vi "MegaAwesome_9_12_12a_JW.vi"() -> ()   [LabVIEW 2011]
uses:
  MegaAwesome_States.ctl
  <vilib>/Utility/file.llb/Read From Spreadsheet File (string).vi
  <vilib>/Utility/file.llb/Write To Spreadsheet File (string).vi
panel:
  in  "Slider Min":dbl=5.0
  in  "Slider Max":dbl=5.0
  out "Opj X Axis":string
  out "X Axis Display Type":string
  in  "Index-Sat":dbl=5.0
  in  "Index-Lin":dbl=5.0
  in  "IndexLog-Lin":dbl=5.0
  in  "IndexLog-Sat":dbl=5.0 caption="Num Pts"
  out "Lin Id-Log Used":dbl[](array[numeric])
  out "Lin-Vg Array-Log Used":dbl[](array[numeric])
  out "Total Width":dbl
  in  "New: Comments":string
  out "Save Array":string[][](array[string])
  out "Folder Index":i32 caption="Length"
  out "Sat Id-Used":dbl[](array[numeric])
  out "Sat Vg Array-Used":dbl[](array[numeric])
  out "Vg Array-Log-Used":dbl[](array[numeric])
  out "Sat Id-Log-Used":dbl[](array[numeric])
  out "Lin Id-Used":dbl[](array[numeric])
  out "Lin-Vg Array-Used":dbl[](array[numeric])
  out "Lin Vd":dbl
  out "Recorded Prop":T1
  out "Current State":T2
  in  "Main Tab Control":T3(tab)
  in  "Image Folder":path
  out "Image File":path=path "D:/UserData/Desktop/Jeremy/WFU/Research/Programs/VI mods/Image Not Found.png"
  in  "Transfer File":path
  out "Transfer Folder":path
  out "Fabrication Prop":T4
  in  "Transport ?":bool
  in  "Transfer Plots":T5(tab)=enum."Saturation"
  in  "Lin-Trans Slider":dbl(slide) step=1.0 scale=-40.0..40.0 scale format="%#_1p"
  out "Sqrt-Lin":cluster{dbl[], dbl[]}[](graph)
  in  "Sat-Trans Slider":dbl(slide) step=1.0 scale=-40.0..40.0 scale format="%#_1p"
  out "Sqrt-Sat":cluster{dbl[], dbl[]}[](graph)
  out "Raw- Lin":cluster{dbl[], dbl[]}[](graph)
  out "Raw- Sat":cluster{dbl[], dbl[]}[](graph)
  in  "Log Plots":enum32{"Linear", "Saturation", "Transport"}(tab)=enum."Saturation"
  in  "Lin-Log Slider":dbl(slide) step=1.0 scale=-40.0..40.0 scale format="%#_1p"
  out "Log-Lin":cluster{dbl[], dbl[]}[](graph)
  in  "Sat-Log Slider":dbl(slide) step=1.0 scale=-40.0..40.0 scale format="%#_1p"
  out "Sat-Log":cluster{dbl[], dbl[]}[](graph)
  out "Transport":cluster{dbl[], dbl[]}[](graph)
  in  "Manual Controls":T6
  in  "File Controls":T7
  out "Date Recorded":string="Date Recorded" caption="Measured"
  out "Data Name:":string
  out "Image Name":string
  out "Index":string
  out "Date Created":string caption="Fabricated"
  in  "Comments:":string
  out "Rec: Length":dbl caption="Length" format="%#_3g"
  out "Rec: Width":dbl caption="Width" format="%#_4g"
  out "Rec: Dielectric (d)":dbl caption="Dielectric (d)" format="%#_3g"
  in  "New: Dielectric":dbl
  in  "New: Length":dbl
  in  "New: Width":dbl
  out "Rec: Temp":dbl caption="Sample Temp" format="%.1f"
  in  "New: Temp":dbl format="%.1f"
  out "Image Out":T8(plugin-control)
  in  "Num Pts":dbl=5.0
  in  "Num Pts Log":dbl=5.0 caption="Num Pts"
  out "Recorded Values Cluster":T9
  out "Calculated Values Cluster":T9 caption="Recorded Values Cluster"
  out "Re-Calculated Values Cluster":T9 caption="Recorded Values Cluster"
  in  "Independant Variable:":string(combo)="Length (um):"
  out "Image Preview":T8(plugin-control)
  in  "No Image File":path=path "\\\\acad1\\physics/Jurchescu-group/JW-PD/Mega Awesome/Image Not Found.png"
  in  "Room Temp":dbl=294.0
  in  "Origin Project File":path=path "\\\\acad1\\physics/Jurchescu-group/JW-PD/Group Library/Origin Project Files/DeviceData_8_10_12a_JW.opj"
  in  "Transport Style Controls":T10={"Transport Line Size"=1, "Transport Line Color"=16772608} {"Transport Line Size" items=["Extra Small", "Small", "Medium", "Large", "Extra Large"]}
  # "Image Location"
  # "Recorded"
  # "Calculated"
  # "Re-Calculated"
  # "Manual"
  # "Used points display at y=0\nValues are wrong w/ slider"
  # "Slider\nDoesn't\nWork"
  # "Slider\nDoesn't\nWork"
  # "No new points displayed"
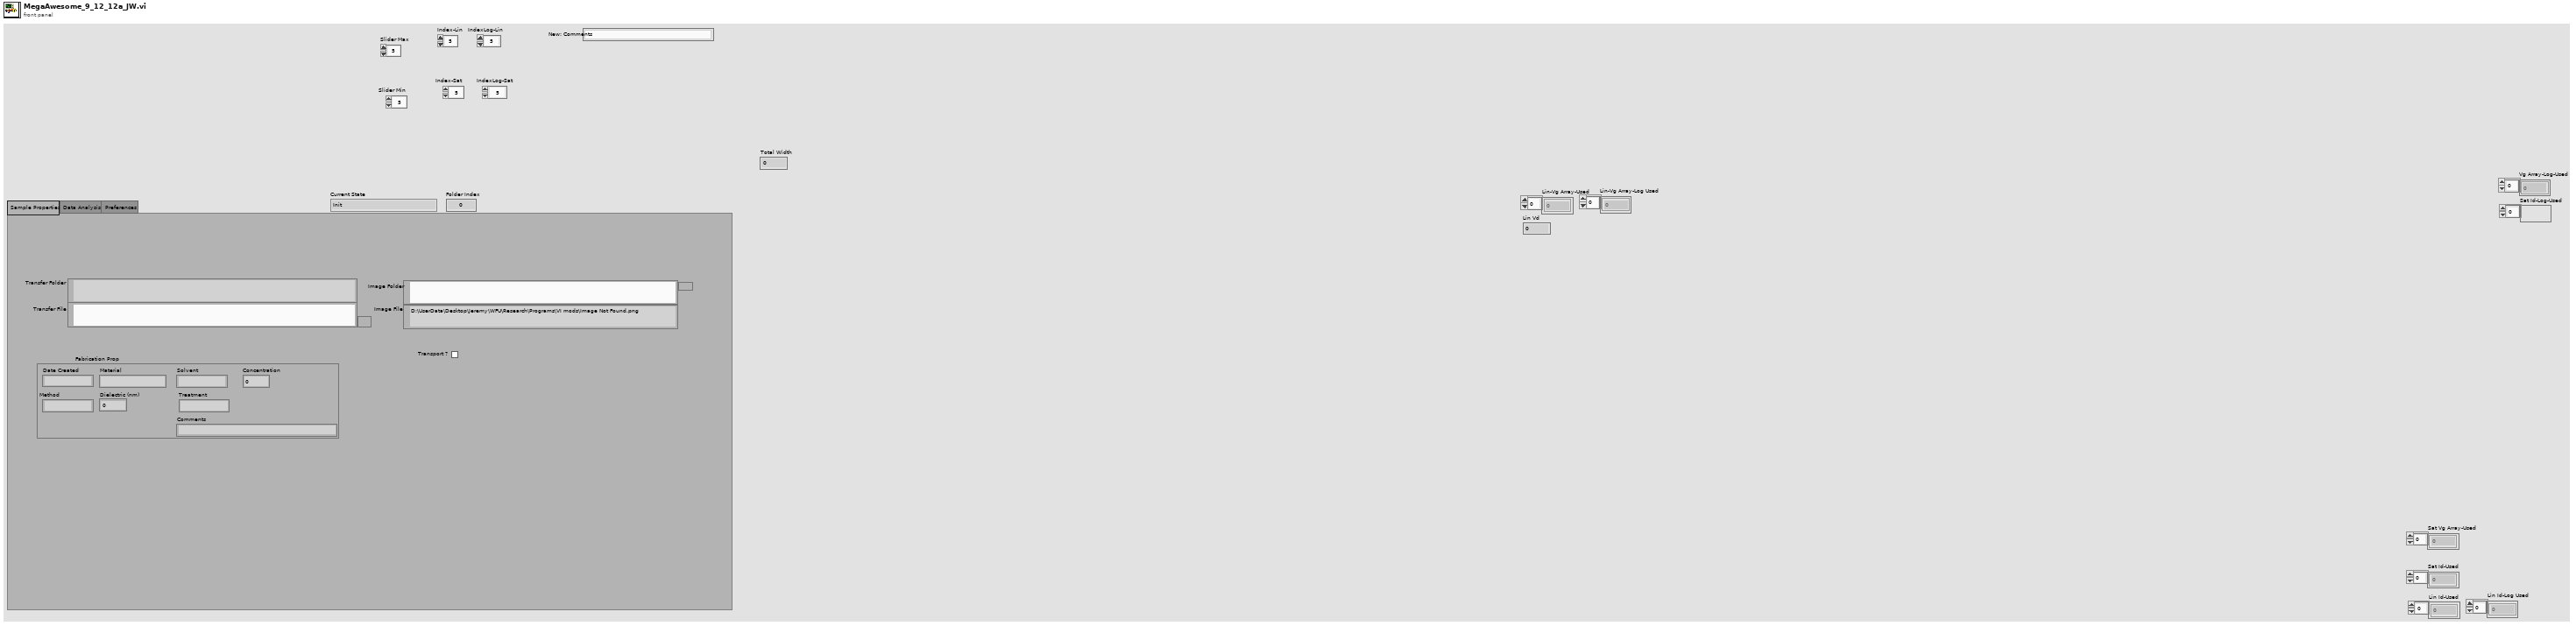
[diagram p1: front panel]
types:
  T1 = cluster{"Date Recorded":string, "Index":string, "Length":dbl, "Width":dbl, "Sample Temp":dbl}
  T2 = typedef "MegaAwesome_States.ctl" = enum16{"Init", "File Missing", "No Event", "Read Data", "Calculated Values", "Re-Calculated Values", "Next File", "Previous File", "Discard File", "Save", "Save Lines", "Export", "Exit"}
  T3 = enum32{"Sample Properties", "Data Analysis", "Preferences"}
  T4 = cluster{"Date Created":string, "Material":string, "Solvent":string, "Concentration":dbl, "Method":string, "Dielectric (nm)":dbl, "Treatment":string, "Comments":string}
  T5 = enum32{"Linear", "Saturation", "Raw-Linear", "Raw-Saturation"}
  T6 = cluster{"Manual-Temp":bool, "Manual-Width":bool, "Manuel-Length":bool, "Manuel-Dielectric":bool, "Manual Comments":bool}
  T7 = cluster{"Previous File":bool, "Discard ":bool, "Save Lines":bool, "Close":bool, "Next File ":bool, "Save":bool, "Save Next":bool, "Export":bool}
  T8 = typedef "IMAQ Image.ctl" = refnum<image>
  T9 = cluster{"Mobility-Sat":dbl, "Moblitity-Lin":dbl, "On/Off":dbl, "Off Current":dbl, "Vt-Sat":dbl, "STS":dbl, "Trap Density-VT":dbl, "Trap Density-STS":dbl}
  T10 = cluster{"Transport Line Size":u16, "Transport Line Color":u32}
  T11 = cluster{"[0]":cluster{dbl[], dbl[]}, "[1]":cluster{dbl[], dbl[]}, "[2]":cluster{dbl[], dbl[]}, "[3]":cluster{dbl[], dbl[]}, "[4]":cluster{dbl[], dbl[]}, "[5]":cluster{dbl[], dbl[]}, "[6]":cluster{dbl[], dbl[]}, "[7]":cluster{dbl[], dbl[]}, "[8]":cluster{dbl[], dbl[]}}
  T12 = cluster{"Sat Vg Used":dbl[], "Sat Sqrt(Id) Used ":dbl[], "Lin Vg Used":dbl[], "Lin Sqrt(Id) Used":dbl[], "Index-Lin":dbl, "Index-Sat":dbl}
  T13 = cluster{"Raw Sat":cluster{dbl[], dbl[]}[], "Sqrt Sat":cluster{dbl[], dbl[]}[], "Log Sat":cluster{dbl[], dbl[]}[], "Raw Lin":cluster{dbl[], dbl[]}[], "Sqrt Lin":cluster{dbl[], dbl[]}[], "Log Lin":cluster{dbl[], dbl[]}[]}
  T14 = cluster{"Mobility-Sat":dbl, "Vt-Sat":dbl, "Mobility-Lin":dbl, "Vt-Lin":dbl, "Off I-Sat":dbl, "On/Off I-Sat":dbl}
  T15 = cluster{"Sat Vg Used":dbl[], "Sat Log(Id) Used":dbl[], "Lin Vg Used":dbl[], "Lin Log(Id) Used":dbl[], "STS Index-Sat":dbl, "STS Index-Lin":dbl}
  T16 = cluster{"Independant  Variable Indicator":string, "Parameter String Indicator":string}
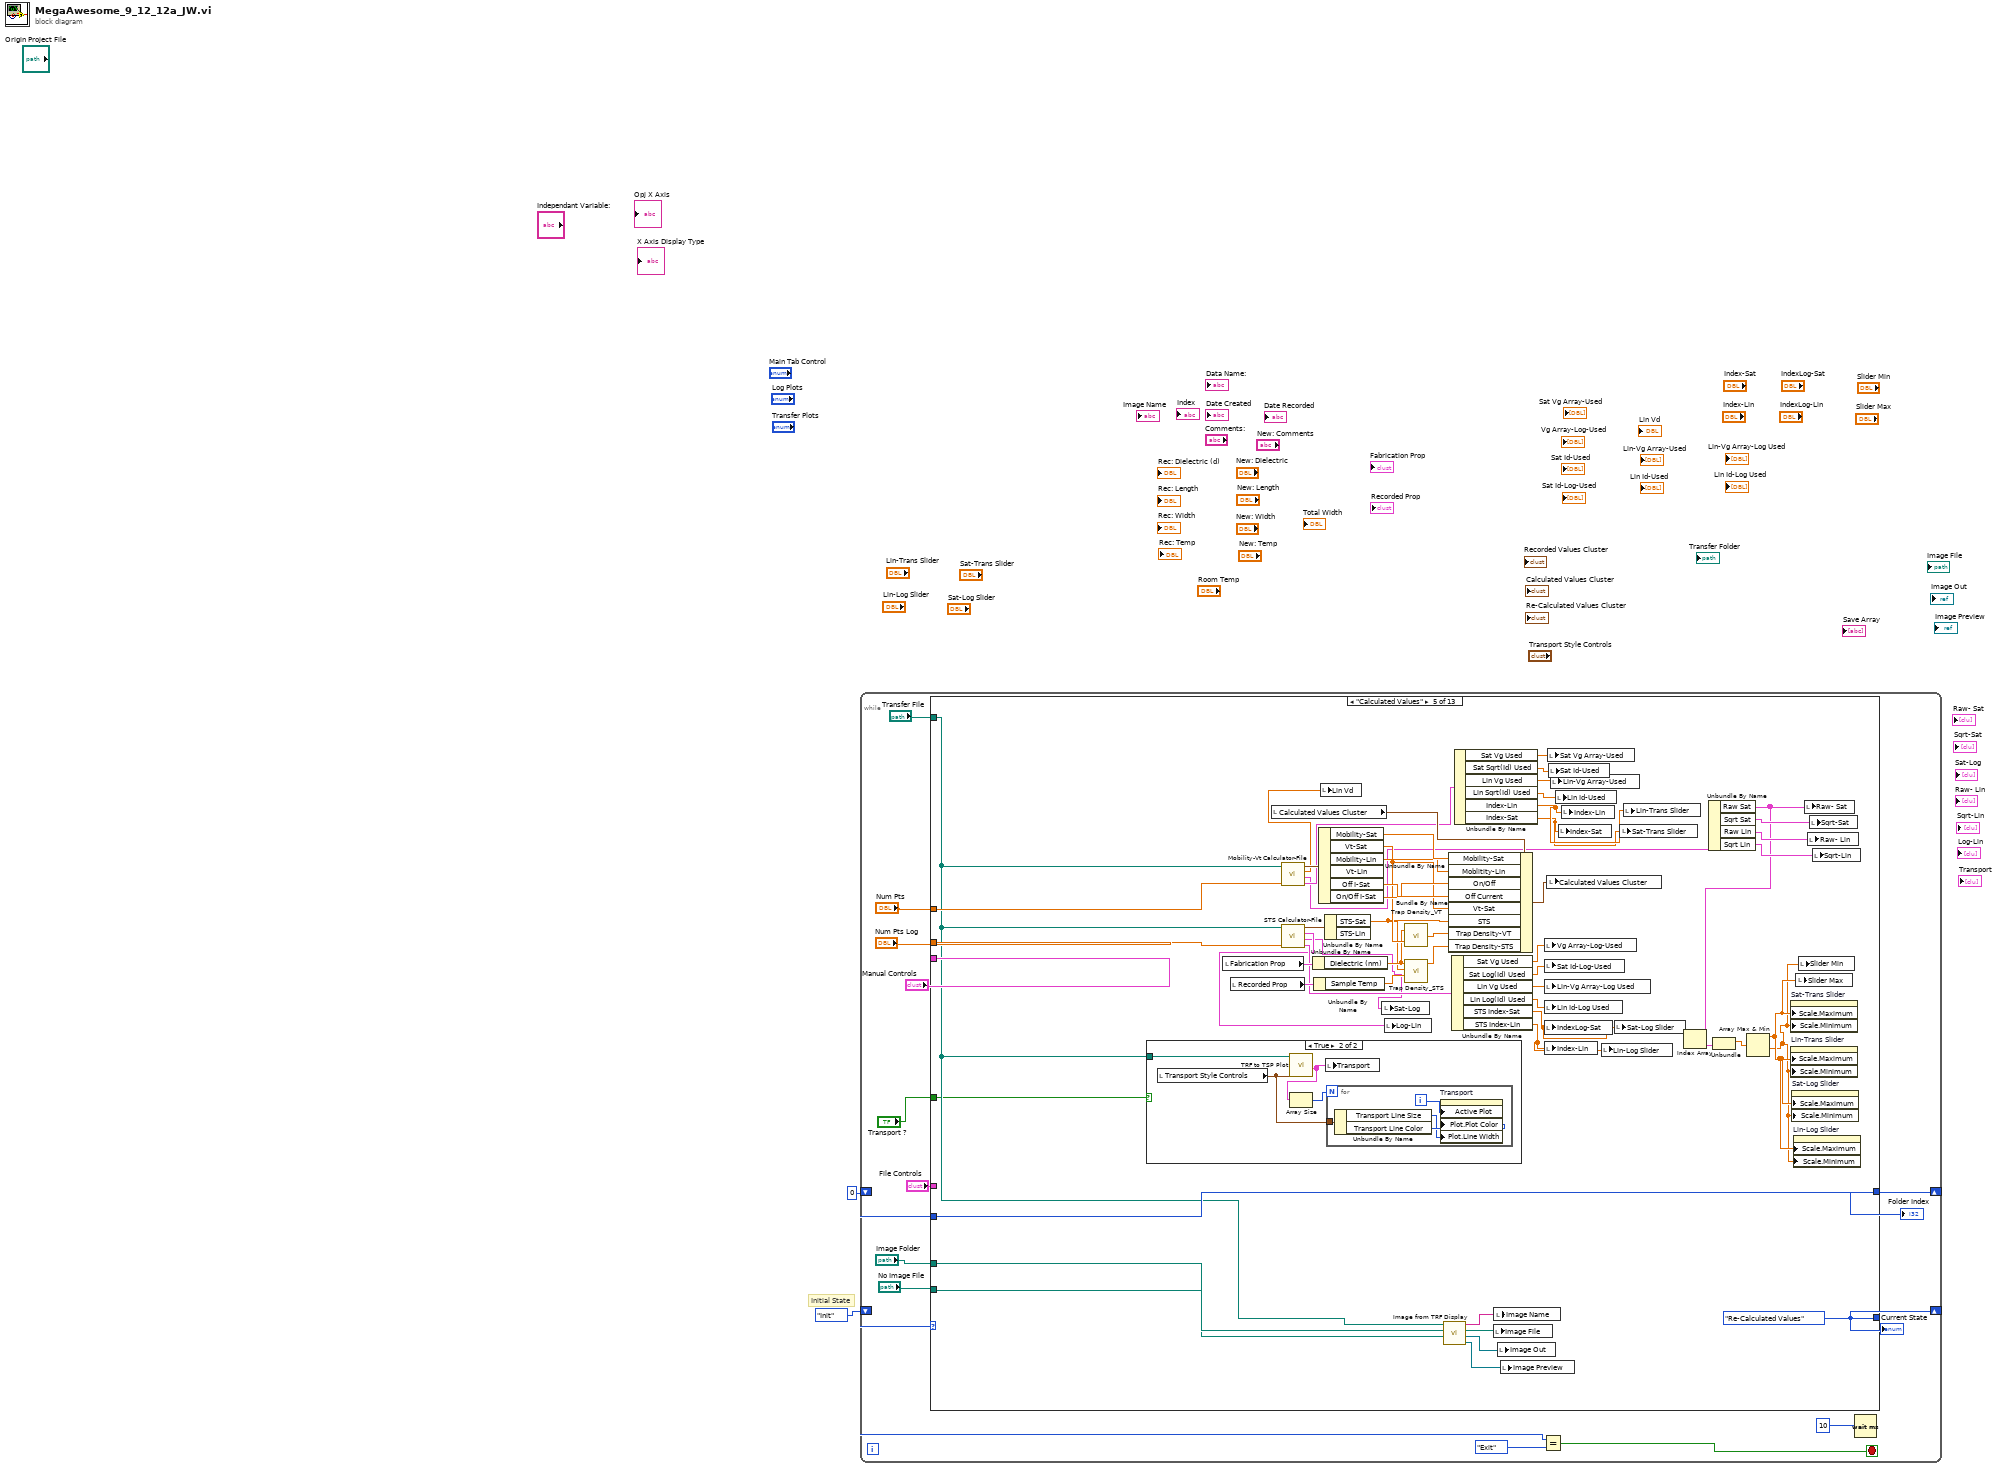
[diagram p0: block diagram]
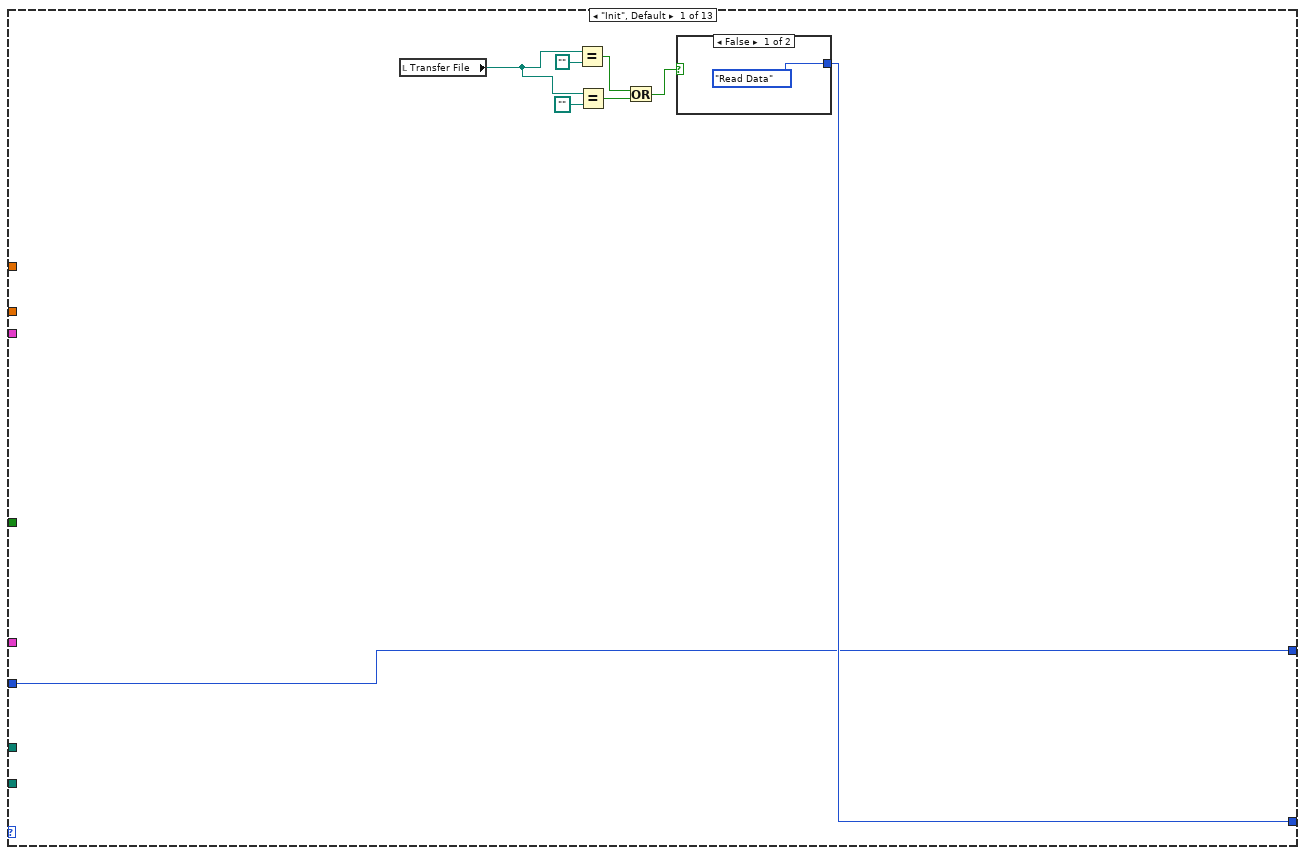
[diagram p2: hidden frame]
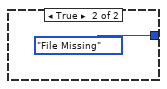
[diagram p3: hidden frame]
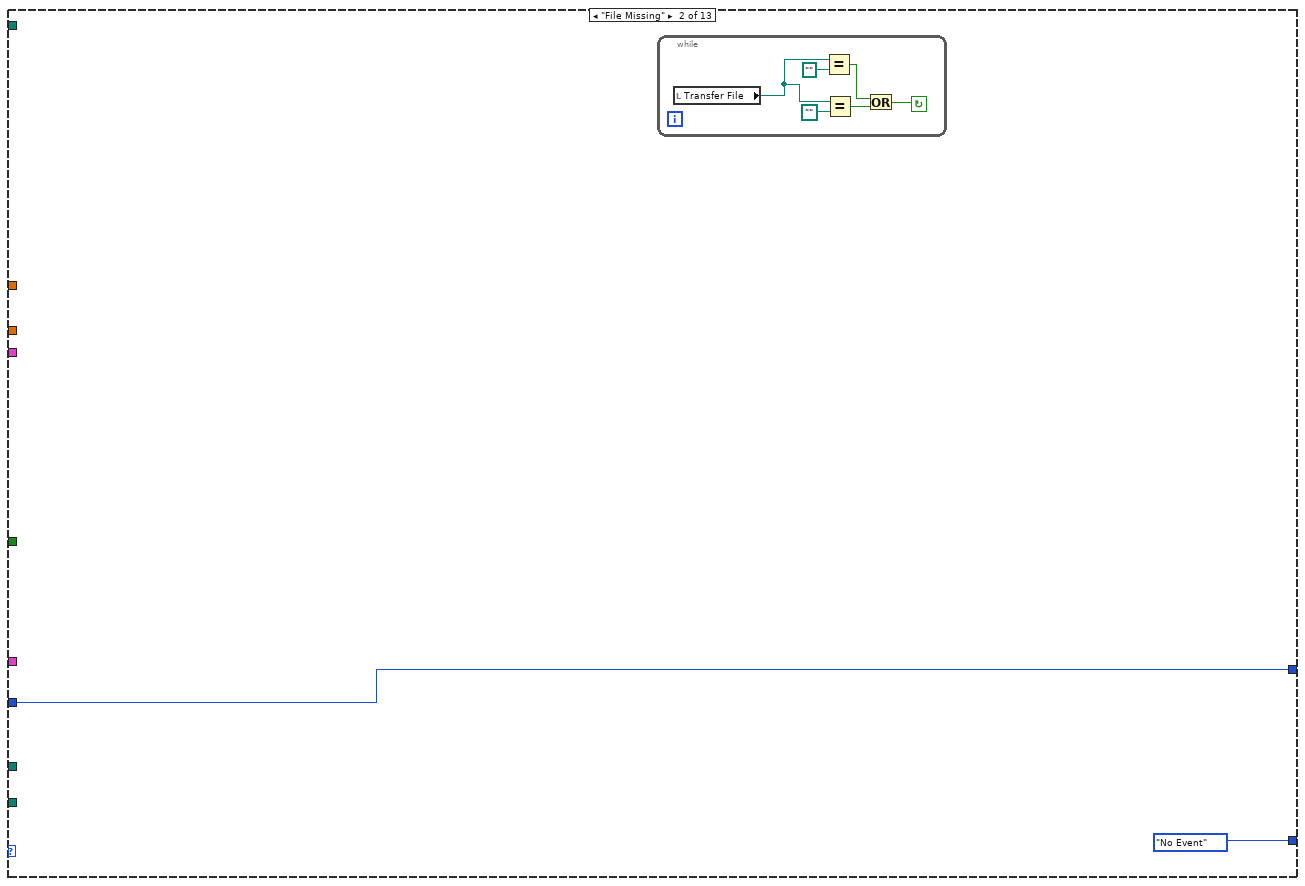
[diagram p4: hidden frame]
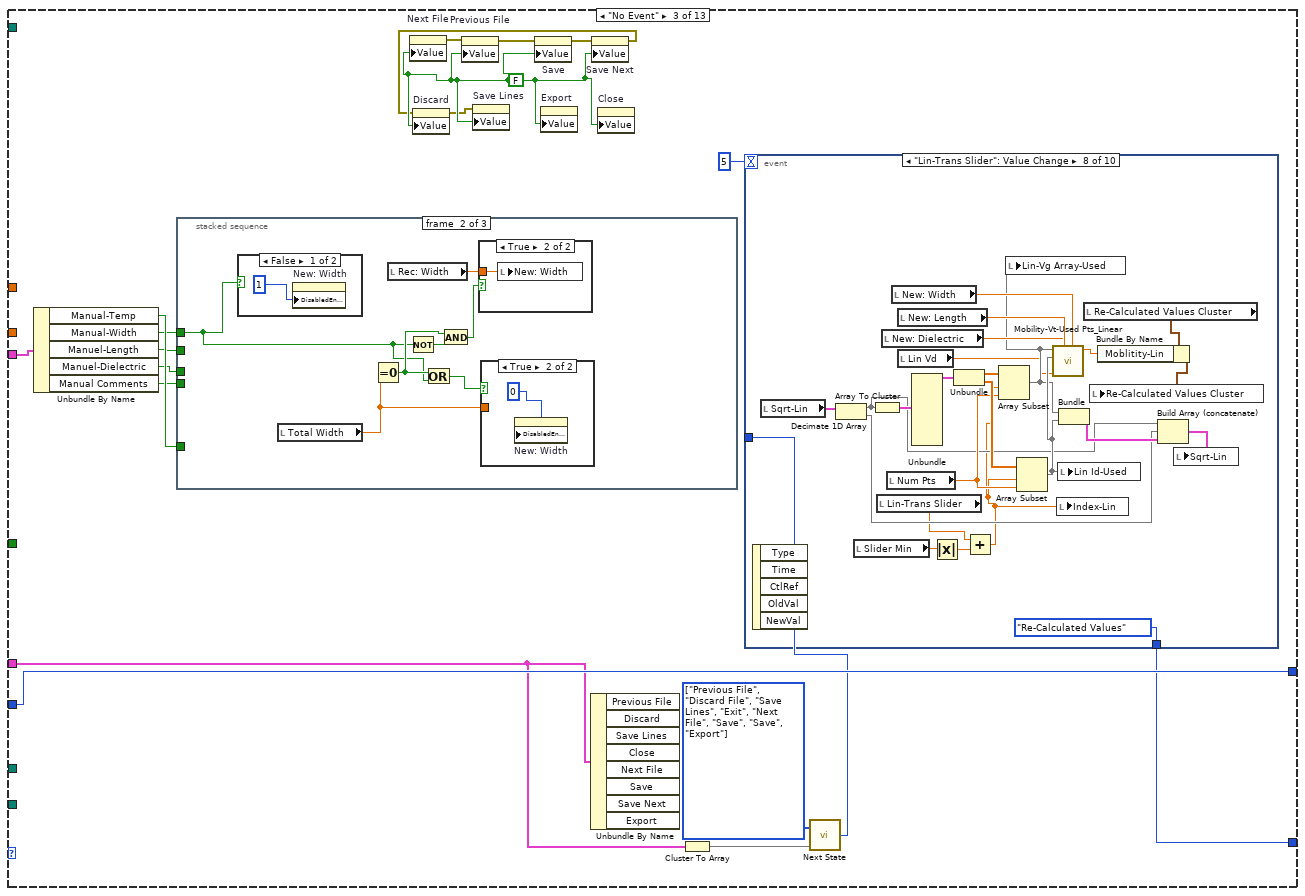
[diagram p5: hidden frame]
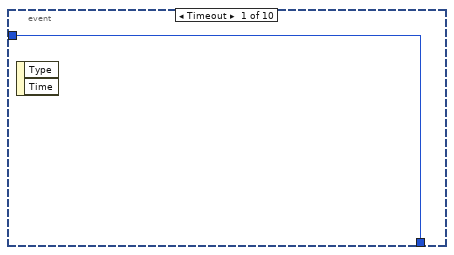
[diagram p6: hidden frame]
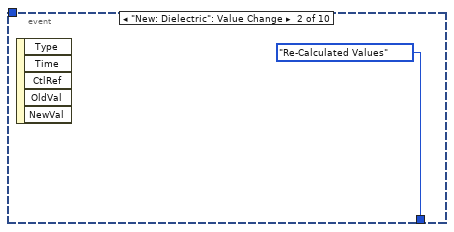
[diagram p7: hidden frame]
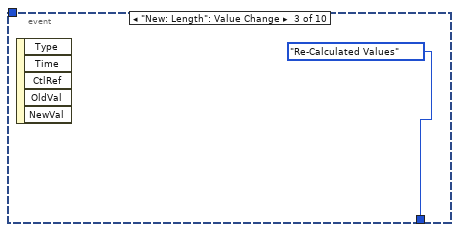
[diagram p8: hidden frame]
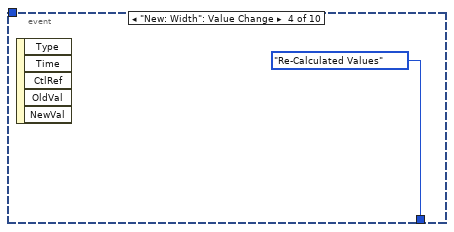
[diagram p9: hidden frame]
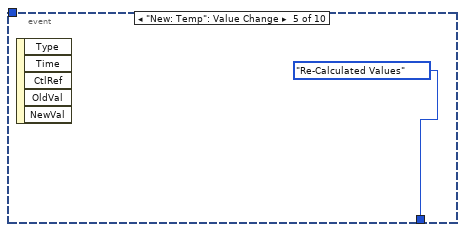
[diagram p10: hidden frame]
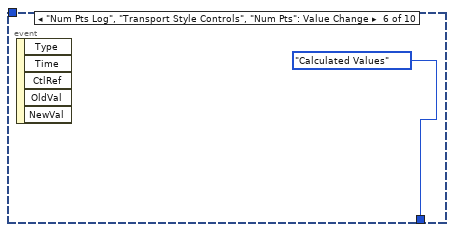
[diagram p11: hidden frame]
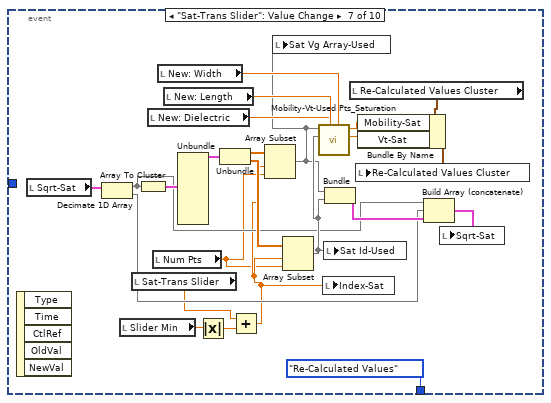
[diagram p12: hidden frame]
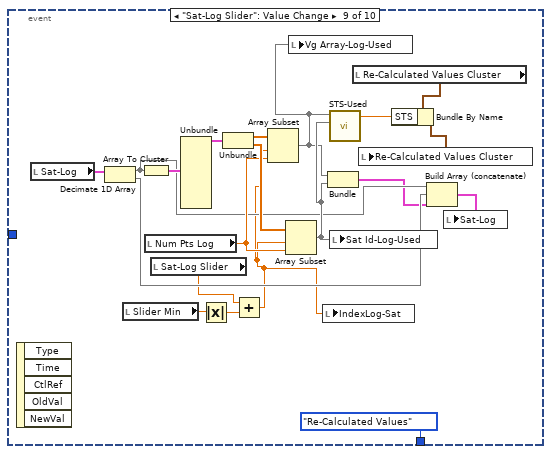
[diagram p13: hidden frame]
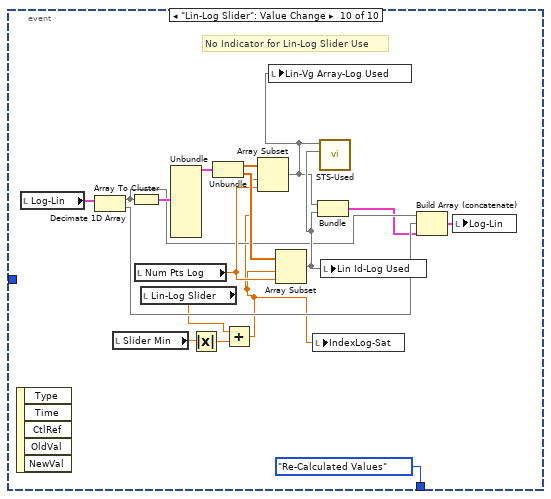
[diagram p14: hidden frame]
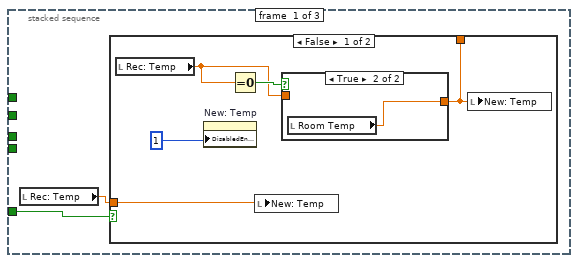
[diagram p15: hidden frame]
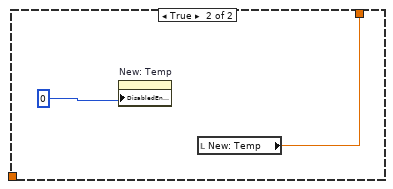
[diagram p17: hidden frame]
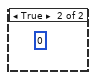
[diagram p18: hidden frame]
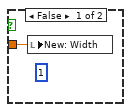
[diagram p20: hidden frame]
diagram:
  # "Initial State"
  n1 = while {
    shift-right: [w14] -> _
    shift-left: MegaAwesome_States."Init" -> [w16]
    shift-right: [w7] -> _
    shift-left: 0 -> [w8]
    stop <- w17 stop-if-true
    n2 = case shown="\"Calculated Values\"" w16 {
      tunnel: [w19 MegaAwesome_States."No Event" w44 MegaAwesome_States."Calculated Values" MegaAwesome_States."Re-Calculated Values" MegaAwesome_States."No Event" MegaAwesome_States."Read Data" MegaAwesome_States."Read Data" MegaAwesome_States."No Event" w344 MegaAwesome_States."No Event" MegaAwesome_States."No Event" MegaAwesome_States."Exit"] -> w14
      tunnel: "Transfer File" -> [_ _ _ w189 w224 _ w313 w325 _ w349 _ _ _]
      tunnel: "Num Pts" -> [_ _ _ _ w248 _ _ _ _ _ _ _ _]
      tunnel: "Num Pts Log" -> [_ _ _ _ w247 _ _ _ _ _ _ _ _]
      tunnel: "Image Folder" -> [_ _ _ _ w244 _ _ _ _ _ _ _ _]
      tunnel: "No Image File" -> [_ _ _ _ w243 _ _ _ _ _ _ _ _]
      tunnel: [w18 w28 w52 w183 w242 w273 w298 w323 w341 w350 w865 w868 w869] -> w7
      tunnel: w8 -> [w18 w28 w52 _ w242 w273 w299 w324 w341 w350 w865 w868 w869]
      tunnel: "Manual Controls" -> [_ _ w46 _ _ _ _ _ _ w348 _ _ _]
      tunnel: "File Controls" -> [_ _ w42 _ _ _ _ _ _ w343 _ _ _]
      tunnel: "Transport ?" -> [_ _ _ _ w210 _ _ _ _ _ _ _ _]
      frame "Init", Default {
        n3 = local read "Transfer File"() -> (w20:path)
        n4 = Equal?(x=w20, y=path "") -> (x = y?=w23:bool)
        n5 = Equal?(x=w20, y=path "") -> (x = y?=w22:bool)
        n6 = Or(x=w23, y=w22) -> (x .or. y?=w25:bool)
        n7 = case shown="False" w25 {
          tunnel: [MegaAwesome_States."Read Data" MegaAwesome_States."File Missing"] -> w19
          frame False {
          }
          frame True {
          }
        }
      }
      frame "File Missing" {
        n8 = while {
          stop <- w30 continue-if-true
          n9 = local read "Transfer File"() -> (w31:path)
          n10 = Equal?(x=w31, y=path "") -> (x = y?=w33:bool)
          n11 = Equal?(x=w31, y=path "") -> (x = y?=w34:bool)
          n12 = Or(x=w33, y=w34) -> (x .or. y?=w30:bool)
        }
      }
      frame "No Event" {
        w41 = FALSE
        w54 = T2[] [enum."Previous File", enum."Discard File", enum."Save Lines", enum."Exit", enum."Next File", enum."Save", enum."Save", enum."Export"] items=["Init", "File Missing", "No Event", "Read Data", "Calculated Values", "Re-Calculated Values", "Next File", "Previous File", "Discard File", "Save", "Save Lines", "Export", "Exit"]
        n13 = Unbundle By Name(w46) -> ("Manual-Temp"=w51:bool, "Manual-Width"=w50:bool, "Manuel-Length"=w49:bool, "Manuel-Dielectric"=w48:bool, "Manual Comments"=w47:bool)
        n14 = stacked-sequence {
          tunnel: w51 -> [w147 _ _]
          tunnel: w50 -> [_ w157 _]
          tunnel: w49 -> [_ _ w172]
          tunnel: w48 -> [_ _ w169]
          tunnel: w47 -> [_ _ w168]
          frame #0 {
            n15 = local read "Rec: Temp"() -> (w146:dbl)
            n16 = case shown="False" w147 {
              tunnel: w146 -> [w152 _]
              tunnel: [w149 w156] -> _
              frame False {
                n17 = local read "Rec: Temp"() -> (w150:dbl)
                n18 = property on="New: Temp" class="DigNum (strict)"("DisabledEnum"=1) -> ()  [unwired: 2 in, 2 out]
                n19 = Equal To 0?(x=w150) -> (x = 0?=w151:bool)
                n20 = local write "New: Temp"(w152) -> ()
                n21 = case shown="True" w151 {
                  tunnel: [w153 w154] -> w149
                  tunnel: w150 -> [w153 _]
                  frame False {
                  }
                  frame True {
                    n22 = local read "Room Temp"() -> (w154:dbl)
                  }
                }
                n23 = local write "New: Temp"(w149) -> ()
              }
              frame True {
                n24 = property on="New: Temp" class="DigNum (strict)"("DisabledEnum"=0) -> ()  [unwired: 2 in, 2 out]
                n25 = local read "New: Temp"() -> (w156:dbl)
              }
            }
          }
          frame #1 {
            n26 = case shown="False" w157 {
              frame False {
                n27 = property on="New: Width" class="DigNum (strict)"("DisabledEnum"=1) -> ()  [unwired: 2 in, 2 out]
              }
              frame True {
                (unwired) 0
              }
            }
            n28 = local read "Total Width"() -> (w163:dbl)
            n29 = Equal To 0?(x=w163) -> (x = 0?=w160:bool)
            n30 = local read "Rec: Width"() -> (w161:dbl)
            n31 = Not(x=w157) -> (.not. x?=w159:bool)
            n32 = Or(x=w160, y=w157) -> (x .or. y?=w162:bool)
            n33 = And(x=w160, y=w159) -> (x .and. y?=w158:bool)
            n34 = case shown="True" w158 {
              tunnel: w161 -> [_ w165]
              frame False {
              }
              frame True {
                n35 = local write "New: Width"(w165) -> ()
              }
            }
            n36 = case shown="True" w162 {
              tunnel: w163 -> [w166 _]
              frame False {
                (unwired) 1
                n37 = local write "New: Width"(w166) -> ()
              }
              frame True {
                n38 = property on="New: Width" class="DigNum (strict)"("DisabledEnum"=0) -> ()  [unwired: 2 in, 2 out]
              }
            }
          }
          frame #2 {
            n39 = local read "Rec: Length"() -> (w173:dbl)
            n40 = case shown="True" w172 {
              tunnel: w173 -> [w181 _]
              frame False {
                n41 = local write "New: Length"(w181) -> ()
                n42 = property on="New: Length" class="DigNum (strict)"("DisabledEnum"=1) -> ()  [unwired: 2 in, 2 out]
              }
              frame True {
                n43 = property on="New: Length" class="DigNum (strict)"("DisabledEnum"=0) -> ()  [unwired: 2 in, 2 out]
              }
            }
            n44 = local read "Comments:"() -> (w170:string)
            n45 = local read "Rec: Dielectric (d)"() -> (w171:dbl)
            n46 = case shown="True" w168 {
              tunnel: w170 -> [w175 _]
              frame False {
                n47 = local write "New: Comments"(w175) -> ()
                n48 = property on="New: Comments" class="Str"("DisabledEnum"=1) -> ()  [unwired: 2 in, 2 out]
              }
              frame True {
                n49 = property on="New: Comments" class="Str"("DisabledEnum"=0) -> ()  [unwired: 2 in, 2 out]
              }
            }
            n50 = case shown="True" w169 {
              tunnel: w171 -> [w178 _]
              frame False {
                n51 = local write "New: Dielectric"(w178) -> ()
                n52 = property on="New: Dielectric" class="DigNum (strict)"("DisabledEnum"=1) -> ()  [unwired: 2 in, 2 out]
              }
              frame True {
                n53 = property on="New: Dielectric" class="DigNum (strict)"("DisabledEnum"=0) -> ()  [unwired: 2 in, 2 out]
              }
            }
          }
        }
        n54 = property on="Next File" class="Bool (strict)"("Value"=w41) -> (error out=w40:errorcluster)  [unwired: 2 in, 1 out]
        n55 = property on="Previous File" class="Bool (strict)"(error in=w40, "Value"=w41) -> (error out=w39:errorcluster)  [unwired: 1 in, 1 out]
        n56 = property on="Save" class="Bool (strict)"(error in=w39, "Value"=w41) -> (error out=w38:errorcluster)  [unwired: 1 in, 1 out]
        n57 = property on="Export" class="Bool (strict)"("Value"=w41) -> ()  [unwired: 2 in, 2 out]
        n58 = Unbundle By Name(w42) -> ()  [unwired: 8 out]
        n59 = property on="Save Next" class="Bool (strict)"(error in=w38, "Value"=w41) -> (error out=w37:errorcluster)  [unwired: 1 in, 1 out]
        n60 = property on="Discard" class="Bool (strict)"(error in=w37, "Value"=w41) -> (error out=w36:errorcluster)  [unwired: 1 in, 1 out]
        n61 = property on="Save Lines" class="Bool (strict)"(error in=w36, "Value"=w41) -> ()  [unwired: 1 in, 2 out]
        n62 = property on="Close" class="Bool (strict)"("Value"=w41) -> ()  [unwired: 2 in, 2 out]
        n63 = Cluster To Array(cluster=w42) -> (array=w53:bool[])
        n64 = call "Next State.vi"("Buttons []"=w53, "States []"=w54) -> ("Enum"=w45:T2)
        n65 = event shown="[7] \"Lin-Trans Slider\": Value Change" {
          selector: _ -> [_ _ _ _ _ _ _ _ _ _]
          dyn-events: _ -> [_ _ _ _ _ _ _ _ _ _]
          timeout: 5 -> [_ _ _ _ _ _ _ _ _ _]
          tunnel: w45 -> [w55 _ _ _ _ _ _ _ _ _]
          tunnel: [w55 MegaAwesome_States."Re-Calculated Values" MegaAwesome_States."Re-Calculated Values" MegaAwesome_States."Re-Calculated Values" MegaAwesome_States."Re-Calculated Values" MegaAwesome_States."Calculated Values" MegaAwesome_States."Re-Calculated Values" MegaAwesome_States."Re-Calculated Values" MegaAwesome_States."Re-Calculated Values" MegaAwesome_States."Re-Calculated Values"] -> w44
          event Timeout {
            n66 = event-data() -> ()  [unwired: 1 in, 2 out]
          }
          event "New: Dielectric": Value Change {
            n67 = event-data() -> ()  [unwired: 1 in, 5 out]
          }
          event "New: Length": Value Change {
            n68 = event-data() -> ()  [unwired: 1 in, 5 out]
          }
          event "New: Width": Value Change {
            n69 = event-data() -> ()  [unwired: 1 in, 5 out]
          }
          event "New: Temp": Value Change {
            n70 = event-data() -> ()  [unwired: 1 in, 5 out]
          }
          event "Num Pts Log", "Transport Style Controls", "Num Pts": Value Change {
            n71 = event-data() -> ()  [unwired: 1 in, 5 out]
          }
          event "Sat-Trans Slider": Value Change {
            n72 = event-data() -> ()  [unwired: 1 in, 5 out]
            n73 = local read "Sqrt-Sat"() -> (w84:cluster{dbl[], dbl[]}[])
            n74 = Decimate 1D Array(w84) -> (w68:cluster{dbl[], dbl[]}[], w69:cluster{dbl[], dbl[]}[])
            n75 = local read "Slider Min"() -> (w65:dbl)
            n76 = local read "Sat-Trans Slider"() -> (w63:dbl)
            n77 = Array To Cluster(array=w68) -> (cluster=w83:T11)
            n78 = local read "New: Dielectric"() -> (w78:dbl)
            n79 = local read "Num Pts"() -> (w61:dbl)
            n80 = local read "New: Width"() -> (w80:dbl)
            n81 = local read "New: Length"() -> (w79:dbl)
            n82 = Unbundle(w83) -> ("[0]"=w82:cluster{dbl[], dbl[]})  [unwired: 8 out]
            n83 = Absolute Value(x=w65) -> (abs(x)=w64:dbl)
            n84 = Unbundle(w82) -> (w66:dbl[], w81:dbl[])
            n85 = Add(x=w63, y=w64) -> (x+y=w62:dbl)
            n86 = Array Subset(array=w66, index=w62, length=w61) -> (w76:dbl[])
            n87 = local write "Sat Vg Array-Used"(w76) -> ()
            n88 = Array Subset(array=w81, index=w62, length=w61) -> (w77:dbl[])
            n89 = call "Mobility-Vt-Used Pts_Saturation.vi"("Width"=w80, "Length"=w79, "Dielectric (d)"=w78, "Sat Id Used"=w77, "Vg Used"=w76) -> ("Vt"=w72:dbl, "Mobility"=w73:dbl)  [unwired: 4 in, 1 out]
            n90 = local write "Index-Sat"(w62) -> ()
            n91 = local write "Sat Id-Used"(w77) -> ()
            n92 = Bundle(w76, w77) -> (w70:cluster{dbl[], dbl[]})  [unwired: 1 in]
            n93 = local read "Re-Calculated Values Cluster"() -> (w75:T9)
            n94 = Bundle By Name(cluster=w75, "Mobility-Sat"=w73, "Vt-Sat"=w72) -> (w74:T9)
            n95 = local write "Re-Calculated Values Cluster"(w74) -> ()
            n96 = Build Array (concatenate)(w68, w69, w70) -> (w67:cluster{dbl[], dbl[]}[])
            n97 = local write "Sqrt-Sat"(w67) -> ()
          }
          event "Lin-Trans Slider": Value Change {
            n98 = event-data() -> ()  [unwired: 1 in, 5 out]
            n99 = local read "Sqrt-Lin"() -> (w108:cluster{dbl[], dbl[]}[])
            n100 = Decimate 1D Array(w108) -> (w93:cluster{dbl[], dbl[]}[], w94:cluster{dbl[], dbl[]}[])
            n101 = local read "Slider Min"() -> (w90:dbl)
            n102 = Array To Cluster(array=w93) -> (cluster=w107:T11)
            n103 = local read "Lin-Trans Slider"() -> (w88:dbl)
            n104 = local read "New: Dielectric"() -> (w101:dbl)
            n105 = local read "Num Pts"() -> (w104:dbl)
            n106 = local read "New: Width"() -> (w103:dbl)
            n107 = local read "New: Length"() -> (w102:dbl)
            n108 = local read "Lin Vd"() -> (w85:dbl)
            n109 = Unbundle(w107) -> ("[0]"=w106:cluster{dbl[], dbl[]})  [unwired: 8 out]
            n110 = Absolute Value(x=w90) -> (abs(x)=w89:dbl)
            n111 = Unbundle(w106) -> (w91:dbl[], w105:dbl[])
            n112 = Add(x=w88, y=w89) -> (x+y=w87:dbl)
            n113 = Array Subset(array=w91, index=w87, length=w104) -> (w99:dbl[])
            n114 = local write "Lin-Vg Array-Used"(w99) -> ()
            n115 = Array Subset(array=w105, index=w87, length=w104) -> (w100:dbl[])
            n116 = call "Mobility-Vt-Used Pts_Linear.vi"("Width"=w103, "Length"=w102, "Vd"=w85, "Dielectric (d)"=w101, "Id Used"=w100, "Vg Used"=w99) -> ("Mobility"=w96:dbl)  [unwired: 3 in, 2 out]
            n117 = local write "Index-Lin"(w87) -> ()
            n118 = local write "Lin Id-Used"(w100) -> ()
            n119 = Bundle(w99, w100) -> (w95:cluster{dbl[], dbl[]})  [unwired: 1 in]
            n120 = local read "Re-Calculated Values Cluster"() -> (w98:T9)
            n121 = Bundle By Name(cluster=w98, "Moblitity-Lin"=w96) -> (w97:T9)
            n122 = local write "Re-Calculated Values Cluster"(w97) -> ()
            n123 = Build Array (concatenate)(w93, w94, w95) -> (w92:cluster{dbl[], dbl[]}[])
            n124 = local write "Sqrt-Lin"(w92) -> ()
          }
          event "Sat-Log Slider": Value Change {
            n125 = event-data() -> ()  [unwired: 1 in, 5 out]
            n126 = local read "Sat-Log"() -> (w111:cluster{dbl[], dbl[]}[])
            n127 = Decimate 1D Array(w111) -> (w118:cluster{dbl[], dbl[]}[], w119:cluster{dbl[], dbl[]}[])
            n128 = local read "Slider Min"() -> (w115:dbl)
            n129 = Array To Cluster(array=w118) -> (cluster=w128:T11)
            n130 = local read "Num Pts Log"() -> (w125:dbl)
            n131 = local read "Sat-Log Slider"() -> (w113:dbl)
            n132 = Unbundle(w128) -> ("[0]"=w127:cluster{dbl[], dbl[]})  [unwired: 8 out]
            n133 = Absolute Value(x=w115) -> (abs(x)=w114:dbl)
            n134 = Unbundle(w127) -> (w116:dbl[], w126:dbl[])
            n135 = Add(x=w113, y=w114) -> (x+y=w110:dbl)
            n136 = Array Subset(array=w116, index=w110, length=w125) -> (w123:dbl[])
            n137 = Array Subset(array=w126, index=w110, length=w125) -> (w124:dbl[])
            n138 = local write "Vg Array-Log-Used"(w123) -> ()
            n139 = local write "IndexLog-Sat"(w110) -> ()
            n140 = Bundle(w123, w124) -> (w109:cluster{dbl[], dbl[]})  [unwired: 1 in]
            n141 = call "STS-Used.vi"("Id Used"=w124, "Vg-Used"=w123) -> ("STS"=w120:dbl)  [unwired: 9 in]
            n142 = local write "Sat Id-Log-Used"(w124) -> ()
            n143 = local read "Re-Calculated Values Cluster"() -> (w122:T9)
            n144 = Bundle By Name(cluster=w122, "STS"=w120) -> (w121:T9)
            n145 = local write "Re-Calculated Values Cluster"(w121) -> ()
            n146 = Build Array (concatenate)(w118, w119, w109) -> (w117:cluster{dbl[], dbl[]}[])
            n147 = local write "Sat-Log"(w117) -> ()
          }
          event "Lin-Log Slider": Value Change {
            # "No Indicator for Lin-Log Slider Use"
            n148 = event-data() -> ()  [unwired: 1 in, 5 out]
            n149 = local read "Log-Lin"() -> (w132:cluster{dbl[], dbl[]}[])
            n150 = Decimate 1D Array(w132) -> (w138:cluster{dbl[], dbl[]}[], w139:cluster{dbl[], dbl[]}[])
            n151 = local read "Slider Min"() -> (w135:dbl)
            n152 = Array To Cluster(array=w138) -> (cluster=w145:T11)
            n153 = local read "Num Pts Log"() -> (w142:dbl)
            n154 = local read "Lin-Log Slider"() -> (w133:dbl)
            n155 = Unbundle(w145) -> ("[0]"=w144:cluster{dbl[], dbl[]})  [unwired: 8 out]
            n156 = Absolute Value(x=w135) -> (abs(x)=w134:dbl)
            n157 = Unbundle(w144) -> (w136:dbl[], w143:dbl[])
            n158 = Add(x=w133, y=w134) -> (x+y=w131:dbl)
            n159 = Array Subset(array=w136, index=w131, length=w142) -> (w140:dbl[])
            n160 = local write "Lin-Vg Array-Log Used"(w140) -> ()
            n161 = Array Subset(array=w143, index=w131, length=w142) -> (w141:dbl[])
            n162 = local write "IndexLog-Sat"(w131) -> ()
            n163 = Bundle(w140, w141) -> (w130:cluster{dbl[], dbl[]})  [unwired: 1 in]
            n164 = call "STS-Used.vi"("Id Used"=w141, "Vg-Used"=w140) -> ()  [unwired: 9 in, 1 out]
            n165 = local write "Lin Id-Log Used"(w141) -> ()
            n166 = Build Array (concatenate)(w138, w139, w130) -> (w137:cluster{dbl[], dbl[]}[])
            n167 = local write "Log-Lin"(w137) -> ()
          }
        }
      }
      frame "Read Data" {
        n168 = call "Recorded Values.vi"("Path"=w189) -> ("Recorded Char"=w207:T9, "Recorded Prop"=w197:T1, "Fabrication Prop"=w191:T4)  [unwired: 8 in]
        n169 = Strip Path(path=w189) -> (stripped path=w190:path, name=w188:string)
        n170 = local write "Fabrication Prop"(w191) -> ()
        n171 = local write "Recorded Prop"(w197) -> ()
        n172 = Unbundle By Name(w197) -> ("Date Recorded"=w196:string, "Index"=w194:string, "Length"=w195:dbl, "Width"=w193:dbl, "Sample Temp"=w192:dbl)
        n173 = local write "Recorded Values Cluster"(w207) -> ()
        n174 = Unbundle By Name(w197) -> ("Sample Temp"=w200:dbl)
        n175 = Unbundle By Name(w191) -> ("Dielectric (nm)"=w185:dbl, "Comments"=w184:string)
        n176 = List Folder(path=w190) -> (filenames=w186:string[])  [unwired: 3 in, 3 out]
        n177 = local write "Rec: Dielectric (d)"(w185) -> ()
        n178 = local write "Date Created"(w196) -> ()
        n179 = local write "Index"(w194) -> ()
        n180 = local write "Rec: Length"(w195) -> ()
        n181 = local write "Rec: Width"(w193) -> ()
        n182 = local write "Rec: Temp"(w192) -> ()
        n183 = Equal To 0?(x=w200) -> (x = 0?=w203:bool)
        n184 = Number To Decimal String(number=w200) -> (decimal integer string=w204:string)  [unwired: 1 in]
        n185 = local write "Comments:"(w184) -> ()
        n186 = Search 1D Array(1D array=w186, element=w188) -> (index of element=w183:i32)  [unwired: 1 in]
        n187 = Equal?(x="", y=w204) -> (x = y?=w202:bool)
        n188 = Index Array(array=w186, index=w183) -> (element=w187:string)
        n189 = Or(x=w203, y=w202) -> (x .or. y?=w201:bool)
        n190 = local write "Data Name:"(w187) -> ()
        n191 = case shown="False" w201 {
          tunnel: [w208 w209] -> w198
          tunnel: w200 -> [w208 _]
          frame False {
          }
          frame True {
            n192 = local read "Room Temp"() -> (w209:dbl)
          }
        }
        n193 = local write "New: Temp"(w198) -> ()
        n194 = Bundle By Name(cluster=w197, "Sample Temp"=w198) -> (w199:T1)
        n195 = local write "Recorded Prop"(w199) -> ()
      }
      frame "Calculated Values" {
        n196 = case shown="True" w210 {
          tunnel: w224 -> [_ w267]
          frame False {
          }
          frame True {
            n197 = local read "Transport Style Controls"() -> (w266:T10)
            n198 = call "TRF to TSP Plot.vi"("Transport Graph Properties"=w266, "Transfer File"=w267) -> ("Transport"=w265:cluster{ext[], ext[]}[])  [unwired: 7 in, 2 out]
            n199 = Array Size(array=w265) -> (size(s)=w264:i32)
            n200 = local write "Transport"(w265) -> ()
            n201 = for {
              N: w264 -> [_]
              tunnel: w266 -> [w271]
              i -> [w270]
              n202 = Unbundle By Name(w271) -> ("Transport Line Size"=w268:u16, "Transport Line Color"=w269:u32)
              n203 = property on="Transport" class="XYGraph (strict)"("Active Plot"=w270, "Plot.Plot Color"=w269, "Plot.Line Width"=w268) -> ()  [unwired: 2 in, 2 out]
            }
          }
        }
        n204 = local read "Fabrication Prop"() -> (w253:T4)
        n205 = local read "Recorded Prop"() -> (w246:T1)
        n206 = local read "Calculated Values Cluster"() -> (w263:T9)
        n207 = call "Mobility-Vt Calculator-File.vi"("NumPts"=w248, "Path"=w224) -> ("Used Points"=w241:T12, "Graph Cluster"=w230:T13, "Lin Vd"=w237:dbl, "Output"=w261:T14)  [unwired: 6 in]
        n208 = call "STS Calculator-File.vi"("NumPts"=w247, "Path"=w224) -> ("Used Points"=w235:T15, "XY Graph-Sat"=w217:cluster{dbl[], dbl[]}[], "XY Graph-Lin"=w218:cluster{dbl[], dbl[]}[], "Ouput"=w256:cluster{"STS-Sat":dbl, "STS-Lin":dbl})  [unwired: 6 in]
        n209 = Unbundle By Name(w253) -> ("Dielectric (nm)"=w251:dbl)
        n210 = Unbundle By Name(w246) -> ("Sample Temp"=w245:dbl)
        n211 = Unbundle By Name(w261) -> ("Mobility-Sat"=w260:dbl, "Vt-Sat"=w252:dbl, "Mobility-Lin"=w259:dbl, "Off I-Sat"=w258:dbl, "On/Off I-Sat"=w257:dbl)  [unwired: 1 out]
        n212 = local write "Lin Vd"(w237) -> ()
        n213 = Unbundle By Name(w256) -> ("STS-Sat"=w250:dbl)  [unwired: 1 out]
        n214 = local write "Sat-Log"(w217) -> ()
        n215 = local write "Log-Lin"(w218) -> ()
        n216 = call "Trap Density_VT.vi"("VT"=w252, "Dielectric"=w251) -> ("Trap Density-VT"=w255:dbl)
        n217 = call "Trap Density_STS.vi"("Temp (T) [K]"=w245, "S.T.S. (S)"=w250, "Dielectric"=w251) -> ("Trap Density (N)"=w254:dbl)  [unwired: 8 in]
        n218 = call "Image from TRF Display.vi"("No Image File"=w243, "Image Folder"=w244, "Transfer File"=w224) -> ("Image Out 2"=w211:T8, "Image Out"=w212:T8, "Image File"=w213:path, "Image Name"=w214:string)  [unwired: 5 in]
        n219 = Bundle By Name(cluster=w263, "Mobility-Sat"=w260, "Moblitity-Lin"=w259, "On/Off"=w257, "Off Current"=w258, "Vt-Sat"=w252, "STS"=w250, "Trap Density-VT"=w255, "Trap Density-STS"=w254) -> (w262:T9)
        n220 = Unbundle By Name(w235) -> ("Sat Vg Used"=w234:dbl[], "Sat Log(Id) Used"=w233:dbl[], "Lin Vg Used"=w232:dbl[], "Lin Log(Id) Used"=w231:dbl[], "STS Index-Sat"=w215:dbl, "STS Index-Lin"=w216:dbl)
        n221 = Unbundle By Name(w241) -> ("Sat Vg Used"=w240:dbl[], "Sat Sqrt(Id) Used"=w239:dbl[], "Lin Vg Used"=w238:dbl[], "Lin Sqrt(Id) Used"=w236:dbl[], "Index-Lin"=w226:dbl, "Index-Sat"=w225:dbl)
        n222 = local write "Image File"(w213) -> ()
        n223 = local write "Image Name"(w214) -> ()
        n224 = local write "Image Out"(w212) -> ()
        n225 = local write "Image Preview"(w211) -> ()
        n226 = local write "Vg Array-Log-Used"(w234) -> ()
        n227 = local write "Sat Id-Log-Used"(w233) -> ()
        n228 = local write "Lin-Vg Array-Log Used"(w232) -> ()
        n229 = local write "Lin Id-Log Used"(w231) -> ()
        n230 = local write "IndexLog-Sat"(w215) -> ()
        n231 = local write "Index-Lin"(w216) -> ()
        n232 = local write "Calculated Values Cluster"(w262) -> ()
        n233 = local write "Sat Vg Array-Used"(w240) -> ()
        n234 = local write "Sat Id-Used"(w239) -> ()
        n235 = local write "Lin-Vg Array-Used"(w238) -> ()
        n236 = local write "Lin Id-Used"(w236) -> ()
        n237 = local write "Index-Sat"(w225) -> ()
        n238 = local write "Index-Lin"(w226) -> ()
        n239 = local write "Lin-Log Slider"(w216) -> ()
        n240 = local write "Sat-Log Slider"(w215) -> ()
        n241 = local write "Sat-Trans Slider"(w225) -> ()
        n242 = local write "Lin-Trans Slider"(w226) -> ()
        n243 = Unbundle By Name(w230) -> ("Raw Sat"=w223:cluster{dbl[], dbl[]}[], "Sqrt Sat"=w227:cluster{dbl[], dbl[]}[], "Raw Lin"=w229:cluster{dbl[], dbl[]}[], "Sqrt Lin"=w228:cluster{dbl[], dbl[]}[])
        n244 = Index Array(array=w223) -> (element=w222:cluster{dbl[], dbl[]})  [unwired: 1 in]
        n245 = Unbundle(w222) -> (w221:dbl[])  [unwired: 1 out]
        n246 = Array Max & Min(array=w221) -> (max value=w220:dbl, min value=w219:dbl)  [unwired: 2 out]
        n247 = property on="Sat-Trans Slider" class="Slide (strict)"("Scale.Maximum"=w220, "Scale.Minimum"=w219) -> ()  [unwired: 2 in, 2 out]
        n248 = property on="Lin-Trans Slider" class="Slide (strict)"("Scale.Maximum"=w220, "Scale.Minimum"=w219) -> ()  [unwired: 2 in, 2 out]
        n249 = property on="Sat-Log Slider" class="Slide (strict)"("Scale.Maximum"=w220, "Scale.Minimum"=w219) -> ()  [unwired: 2 in, 2 out]
        n250 = property on="Lin-Log Slider" class="Slide (strict)"("Scale.Maximum"=w220, "Scale.Minimum"=w219) -> ()  [unwired: 2 in, 2 out]
        n251 = local write "Slider Max"(w220) -> ()
        n252 = local write "Slider Min"(w219) -> ()
        n253 = local write "Raw- Sat"(w223) -> ()
        n254 = local write "Raw- Lin"(w229) -> ()
        n255 = local write "Sqrt-Sat"(w227) -> ()
        n256 = local write "Sqrt-Lin"(w228) -> ()
      }
      frame "Re-Calculated Values" {
        n257 = local read "Vg Array-Log-Used"() -> (w280:dbl[])
        n258 = local read "Sat Vg Array-Used"() -> (w288:dbl[])
        n259 = local read "Lin-Vg Array-Used"() -> (w294:dbl[])
        n260 = local read "Sat Id-Log-Used"() -> (w279:dbl[])
        n261 = local read "New: Dielectric"() -> (w292:dbl)
        n262 = local read "New: Dielectric"() -> (w277:dbl)
        n263 = local read "New: Length"() -> (w291:dbl)
        n264 = local read "New: Length"() -> (w287:dbl)
        n265 = local read "New: Width"() -> (w290:dbl)
        n266 = local read "New: Width"() -> (w286:dbl)
        n267 = local read "Lin Id-Used"() -> (w293:dbl[])
        n268 = local read "Sat Id-Used"() -> (w285:dbl[])
        n269 = local read "Re-Calculated Values Cluster"() -> (w296:T9)
        n270 = local read "New: Dielectric"() -> (w276:dbl)
        n271 = local read "New: Temp"() -> (w275:dbl)
        n272 = local read "Lin Vd"() -> (w272:dbl)
        n273 = call "Mobility-Vt-Used Pts_Saturation.vi"("Width"=w286, "Length"=w287, "Dielectric (d)"=w277, "Sat Id Used"=w285, "Vg Used"=w288) -> ("Vt"=w283:dbl, "Mobility"=w284:dbl)  [unwired: 4 in, 1 out]
        n274 = call "STS-Used.vi"("Id Used"=w279, "Vg-Used"=w280) -> ("STS"=w278:dbl)  [unwired: 9 in]
        n275 = call "Mobility-Vt-Used Pts_Linear.vi"("Width"=w290, "Length"=w291, "Vd"=w272, "Dielectric (d)"=w292, "Id Used"=w293, "Vg Used"=w294) -> ("Mobility"=w289:dbl)  [unwired: 3 in, 2 out]
        n276 = call "Trap Density_VT.vi"("VT"=w283, "Dielectric"=w277) -> ("Trap Density-VT"=w282:dbl)
        n277 = call "Trap Density_STS.vi"("Temp (T) [K]"=w275, "S.T.S. (S)"=w278, "Dielectric"=w276) -> ("Trap Density (N)"=w274:dbl)  [unwired: 8 in]
        n278 = Bundle By Name(cluster=w296, "Mobility-Sat"=w284, "Moblitity-Lin"=w289, "Vt-Sat"=w283, "STS"=w278, "Trap Density-VT"=w282, "Trap Density-STS"=w274) -> (w295:T9)
        n279 = local write "Re-Calculated Values Cluster"(w295) -> ()
      }
      frame "Next File" {
        n280 = Strip Path(path=w313) -> (stripped path=w303:path, name=w311:string)
        n281 = local write "Transfer Folder"(w303) -> ()
        n282 = List Folder(path=w303) -> (filenames=w297:string[], error out=w306:errorcluster)  [unwired: 3 in, 2 out]
        n283 = Array Size(array=w297) -> (size(s)=w310:i32)
        n284 = Search 1D Array(1D array=w297, element=w311) -> (index of element=w308:i32)  [unwired: 1 in]
        n285 = Decrement(x=w310) -> (x-1=w309:i32)
        n286 = Equal?(x=w309, y=w308) -> (x = y?=w307:bool)
        n287 = case shown="False" w307 {
          tunnel: w299 -> [w316 _]
          tunnel: [w315 0] -> w298
          tunnel: w306 -> [w314 w317]
          tunnel: [w314 w317] -> _
          frame False {
            n288 = Increment(x=w316) -> (x+1=w315:i32)
          }
          frame True {
          }
        }
        n289 = Path To String(path=w303) -> (string=w304:string)
        n290 = Index Array(array=w297, index=w298) -> (element=w305:string)
        n291 = Concatenate Strings(w304, "\\", w305) -> (w301:string)
        n292 = String To Path(string=w301) -> (path=w300:path)
        n293 = local write "Transfer File"(w300) -> ()
      }
      frame "Previous File" {
        n294 = Strip Path(path=w325) -> (stripped path=w322:path, name=w334:string)
        n295 = local write "Transfer Folder"(w322) -> ()
        n296 = List Folder(path=w322) -> (filenames=w326:string[], error out=w331:errorcluster)  [unwired: 3 in, 2 out]
        n297 = Array Size(array=w326) -> (size(s)=w320:i32)
        n298 = Search 1D Array(1D array=w326, element=w334) -> (index of element=w333:i32)  [unwired: 1 in]
        n299 = Decrement(x=w320) -> (x-1=w319:i32)
        n300 = Equal To 0?(x=w333) -> (x = 0?=w332:bool)
        n301 = case shown="False" w332 {
          tunnel: w324 -> [w338 _]
          tunnel: [w337 w339] -> w323
          tunnel: w331 -> [w336 w340]
          tunnel: [w336 w340] -> _
          tunnel: w319 -> [_ w339]
          frame False {
            n302 = Decrement(x=w338) -> (x-1=w337:i32)
          }
          frame True {
          }
        }
        n303 = Path To String(path=w322) -> (string=w321:string)
        n304 = Index Array(array=w326, index=w323) -> (element=w330:string)
        n305 = Concatenate Strings(w321, "\\", w330) -> (w328:string)
        n306 = String To Path(string=w328) -> (path=w327:path)
        n307 = local write "Transfer File"(w327) -> ()
      }
      frame "Discard File" {
      }
      frame "Save" {
        n308 = stacked-sequence {
          seq-local: [w358 _] -> [_ w855]
          seq-local: [w357 _] -> [_ w853]
          tunnel: w349 -> [w359 w856]
          frame #0 {
            # "Saves each Re-calculated parameter in sequence"
            n309 = stacked-sequence {
              tunnel: [_ _ _ _ _ _ _ _ _ _ _ _ _ w823] -> w357
              tunnel: w359 -> [w379 _ _ _ _ _ _ _ _ _ _ _ _ _]
              frame #0 {
                n310 = call-poly <vilib>:"Read From Spreadsheet File.vi"("file path (dialog if empty)"=w379) -> ("all rows"=w378:string[][])  [unwired: 6 in, 4 out]
                n311 = Array Size(array=w378) -> (size(s)=w383:i32[])
                n312 = Array Subset(array=w378, index (row)=0, index (col)=0, length (col)=3) -> (w387:string[][])  [unwired: 1 in]
                n313 = Index Array(array=w383, index=0) -> (element=w381:i32)
                n314 = Reshape Array(w387, w381) -> (w380:string[])
                n315 = Search 1D Array(1D array=w380, element="Dielectric (nm):") -> (index of element=w390:i32)  [unwired: 1 in]
                n316 = Equal?(x=w390, y=-1) -> (x = y?=w389:bool)
                n317 = case shown="False" w389 {
                  tunnel: w378 -> [w398 w402]
                  tunnel: w390 -> [w394 _]
                  tunnel: [w393 w402] -> w388
                  frame False {
                    n318 = local read "Rec: Dielectric (d)"() -> (w400:dbl)
                    n319 = Number To Fractional String(number=w400) -> (F-format string=w395:string)  [unwired: 3 in]
                    n320 = Divide(x=w394, y=3) -> (x/y=w397:dbl)
                    n321 = To Word Integer(number=w397) -> (16bit integer=w396:i16)
                    n322 = Replace Array Subset(array=w398, new element=w395, index (row)=w396, index (col)=1) -> (w393:string[][])
                  }
                  frame True {
                  }
                }
                n323 = local write "Save Array"(w388) -> ()
              }
              frame #1 {
                n324 = local read "Save Array"() -> (w404:string[][])
                n325 = Array Size(array=w404) -> (size(s)=w407:i32[])
                n326 = Array Subset(array=w404, index (row)=0, index (col)=0, length (col)=3) -> (w411:string[][])  [unwired: 1 in]
                n327 = Index Array(array=w407, index=0) -> (element=w405:i32)
                n328 = Reshape Array(w411, w405) -> (w403:string[])
                n329 = Search 1D Array(1D array=w403, element="Comments:") -> (index of element=w414:i32)  [unwired: 1 in]
                n330 = Equal?(x=w414, y=-1) -> (x = y?=w413:bool)
                n331 = case shown="False" w413 {
                  tunnel: w404 -> [w422 w425]
                  tunnel: w414 -> [w419 _]
                  tunnel: [w418 w425] -> w412
                  frame False {
                    n332 = local read "New: Comments"() -> (w417:string)
                    n333 = Divide(x=w419, y=3) -> (x/y=w421:dbl)
                    n334 = To Word Integer(number=w421) -> (16bit integer=w420:i16)
                    n335 = Replace Array Subset(array=w422, new element=w417, index (row)=w420, index (col)=1) -> (w418:string[][])
                  }
                  frame True {
                  }
                }
                n336 = local write "Save Array"(w412) -> ()
              }
              frame #2 {
                n337 = local read "Save Array"() -> (w427:string[][])
                n338 = Array Size(array=w427) -> (size(s)=w430:i32[])
                n339 = Array Subset(array=w427, index (row)=0, index (col)=0, length (col)=3) -> (w434:string[][])  [unwired: 1 in]
                n340 = Index Array(array=w430, index=0) -> (element=w428:i32)
                n341 = Reshape Array(w434, w428) -> (w426:string[])
                n342 = Search 1D Array(1D array=w426, element="Length (um):") -> (index of element=w437:i32)  [unwired: 1 in]
                n343 = Equal?(x=w437, y=-1) -> (x = y?=w436:bool)
                n344 = case shown="False" w436 {
                  tunnel: w427 -> [w447 w450]
                  tunnel: w437 -> [w444 _]
                  tunnel: [w443 w450] -> w435
                  frame False {
                    n345 = local read "New: Length"() -> (w440:dbl)
                    n346 = Divide(x=w444, y=3) -> (x/y=w446:dbl)
                    n347 = Format Value(format string="%#g", value (0)=w440) -> (output string=w441:string)  [unwired: 1 in]
                    n348 = To Word Integer(number=w446) -> (16bit integer=w445:i16)
                    n349 = Replace Array Subset(array=w447, new element=w441, index (row)=w445, index (col)=1) -> (w443:string[][])
                  }
                  frame True {
                  }
                }
                n350 = local write "Save Array"(w435) -> ()
              }
              frame #3 {
                n351 = local read "Save Array"() -> (w452:string[][])
                n352 = Array Size(array=w452) -> (size(s)=w457:i32[])
                n353 = Array Subset(array=w452, index (row)=0, index (col)=0, length (col)=3) -> (w453:string[][])  [unwired: 1 in]
                n354 = Index Array(array=w457, index=0) -> (element=w459:i32)
                n355 = Reshape Array(w453, w459) -> (w451:string[])
                n356 = Search 1D Array(1D array=w451, element="Width (um):") -> (index of element=w462:i32)  [unwired: 1 in]
                n357 = Equal?(x=w462, y=-1) -> (x = y?=w461:bool)
                n358 = case shown="False" w461 {
                  tunnel: w462 -> [w470 _]
                  tunnel: w452 -> [w469 w475]
                  tunnel: [w468 w475] -> w460
                  frame False {
                    n359 = local read "New: Width"() -> (w465:dbl)
                    n360 = Divide(x=w470, y=3) -> (x/y=w472:dbl)
                    n361 = To Word Integer(number=w472) -> (16bit integer=w471:i16)
                    n362 = Format Value(format string="%#g", value (0)=w465) -> (output string=w466:string)  [unwired: 1 in]
                    n363 = Replace Array Subset(array=w469, new element=w466, index (row)=w471, index (col)=1) -> (w468:string[][])
                  }
                  frame True {
                  }
                }
                n364 = local write "Save Array"(w460) -> ()
              }
              frame #4 {
                w485 = "Sample Temp (K):"
                n365 = local read "Save Array"() -> (w477:string[][])
                n366 = Array Size(array=w477) -> (size(s)=w482:i32[])
                n367 = Array Subset(array=w477, index (row)=0, index (col)=0, length (col)=3) -> (w478:string[][])  [unwired: 1 in]
                n368 = Index Array(array=w482, index=0) -> (element=w484:i32)
                n369 = Reshape Array(w478, w484) -> (w476:string[])
                n370 = Search 1D Array(1D array=w476, element=w485) -> (index of element=w488:i32)  [unwired: 1 in]
                n371 = Equal?(x=w488, y=-1) -> (x = y?=w487:bool)
                n372 = case shown="False" w487 {
                  tunnel: w477 -> [w497 w511]
                  tunnel: w488 -> [w494 _]
                  tunnel: [w493 w510] -> w486
                  tunnel: w476 -> [_ w513]
                  tunnel: w485 -> [_ w500]
                  frame False {
                    n373 = local read "New: Temp"() -> (w491:dbl)
                    n374 = Divide(x=w494, y=3) -> (x/y=w496:dbl)
                    n375 = Format Value(format string="%#g", value (0)=w491) -> (output string=w490:string)  [unwired: 1 in]
                    n376 = To Word Integer(number=w496) -> (16bit integer=w495:i16)
                    n377 = Replace Array Subset(array=w497, new element=w490, index (row)=w495, index (col)=1) -> (w493:string[][])
                  }
                  frame True {
                    n378 = local read "New: Temp"() -> (w502:dbl)
                    n379 = Search 1D Array(1D array=w513, element="Width (um):") -> (index of element=w507:i32)  [unwired: 1 in]
                    n380 = Divide(x=w507, y=3) -> (x/y=w508:dbl)
                    n381 = To Word Integer(number=w508) -> (16bit integer=w506:i16)
                    n382 = Format Value(format string="%#g", value (0)=w502) -> (output string=w501:string)  [unwired: 1 in]
                    n383 = Build Array(w500, w501) -> (w504:string[])
                    n384 = Increment(x=w506) -> (x+1=w505:i16)
                    n385 = Insert Into Array(array=w511, index (row)=w505, new element=w504) -> (w510:string[][])  [unwired: 1 in]
                  }
                }
                n386 = local write "Save Array"(w486) -> ()
              }
              frame #5 {
                w523 = "Mobility-Sat (cm^2/Vs):"
                n387 = local read "Save Array"() -> (w515:string[][])
                n388 = Array Size(array=w515) -> (size(s)=w520:i32[])
                n389 = Array Subset(array=w515, index (row)=0, index (col)=0, length (col)=3) -> (w516:string[][])  [unwired: 1 in]
                n390 = Index Array(array=w520, index=0) -> (element=w522:i32)
                n391 = Reshape Array(w516, w522) -> (w514:string[])
                n392 = Search 1D Array(1D array=w514, element=w523) -> (index of element=w526:i32)  [unwired: 1 in]
                n393 = Equal?(x=w526, y=-1) -> (x = y?=w525:bool)
                n394 = case shown="False" w525 {
                  tunnel: w515 -> [w536 w546]
                  tunnel: w526 -> [w533 _]
                  tunnel: [w532 w545] -> w524
                  tunnel: w514 -> [_ w543]
                  tunnel: w523 -> [_ w541]
                  frame False {
                    n395 = local read "Re-Calculated Values Cluster"() -> (w529:T9)
                    n396 = Unbundle By Name(w529) -> ("Mobility-Sat"=w528:dbl)
                    n397 = Divide(x=w533, y=3) -> (x/y=w535:dbl)
                    n398 = To Word Integer(number=w535) -> (16bit integer=w534:i16)
                    n399 = Format Value(format string="%#g", value (0)=w528) -> (output string=w530:string)  [unwired: 1 in]
                    n400 = Replace Array Subset(array=w536, new element=w530, index (row)=w534, index (col)=1) -> (w532:string[][])
                  }
                  frame True {
                    n401 = local read "Re-Calculated Values Cluster"() -> (w540:T9)
                    n402 = Unbundle By Name(w540) -> ("Mobility-Sat"=w539:dbl)
                    n403 = Search 1D Array(1D array=w543, element="Mobility (cm^2/Vs):") -> (index of element=w549:i32)  [unwired: 1 in]
                    n404 = Divide(x=w549, y=3) -> (x/y=w550:dbl)
                    n405 = To Word Integer(number=w550) -> (16bit integer=w542:i16)
                    n406 = Format Value(format string="%#g", value (0)=w539) -> (output string=w544:string)  [unwired: 1 in]
                    n407 = Build Array(w541, w544) -> (w548:string[])
                    n408 = Replace Array Subset(array=w546, new element=w548, index (row)=w542) -> (w545:string[][])  [unwired: 1 in]
                  }
                }
                n409 = local write "Save Array"(w524) -> ()
              }
              frame #6 {
                w562 = "Mobility-Lin (cm^2/Vs):"
                n410 = local read "Save Array"() -> (w553:string[][])
                n411 = Array Size(array=w553) -> (size(s)=w559:i32[])
                n412 = Array Subset(array=w553, index (row)=0, index (col)=0, length (col)=3) -> (w555:string[][])  [unwired: 1 in]
                n413 = Index Array(array=w559, index=0) -> (element=w561:i32)
                n414 = Reshape Array(w555, w561) -> (w554:string[])
                n415 = Search 1D Array(1D array=w554, element=w562) -> (index of element=w565:i32)  [unwired: 1 in]
                n416 = Equal?(x=w565, y=-1) -> (x = y?=w564:bool)
                n417 = case shown="True" w564 {
                  tunnel: w553 -> [w575 w583]
                  tunnel: w565 -> [w572 _]
                  tunnel: [w571 w582] -> w563
                  tunnel: w554 -> [_ w581]
                  tunnel: w562 -> [_ w580]
                  frame False {
                    n418 = local read "Re-Calculated Values Cluster"() -> (w568:T9)
                    n419 = Unbundle By Name(w568) -> ("Moblitity-Lin"=w567:dbl)
                    n420 = Divide(x=w572, y=3) -> (x/y=w574:dbl)
                    n421 = To Word Integer(number=w574) -> (16bit integer=w573:i16)
                    n422 = Format Value(format string="%#g", value (0)=w567) -> (output string=w569:string)  [unwired: 1 in]
                    n423 = Replace Array Subset(array=w575, new element=w569, index (row)=w573, index (col)=1) -> (w571:string[][])
                  }
                  frame True {
                    n424 = local read "Re-Calculated Values Cluster"() -> (w579:T9)
                    n425 = Unbundle By Name(w579) -> ("Moblitity-Lin"=w578:dbl)
                    n426 = Search 1D Array(1D array=w581, element="Mobility-Sat (cm^2/Vs):") -> (index of element=w588:i32)  [unwired: 1 in]
                    n427 = Divide(x=w588, y=3) -> (x/y=w589:dbl)
                    n428 = To Word Integer(number=w589) -> (16bit integer=w587:i16)
                    n429 = Format Value(format string="%#g", value (0)=w578) -> (output string=w592:string)  [unwired: 1 in]
                    n430 = Build Array(w580, w592) -> (w585:string[])
                    n431 = Increment(x=w587) -> (x+1=w586:i16)
                    n432 = Insert Into Array(array=w583, index (row)=w586, new element=w585) -> (w582:string[][])  [unwired: 1 in]
                  }
                }
                n433 = local write "Save Array"(w563) -> ()
              }
              frame #7 {
                w602 = "On/Off I-Sat:"
                n434 = local read "Save Array"() -> (w593:string[][])
                n435 = Array Size(array=w593) -> (size(s)=w599:i32[])
                n436 = Array Subset(array=w593, index (row)=0, index (col)=0, length (col)=3) -> (w595:string[][])  [unwired: 1 in]
                n437 = Index Array(array=w599, index=0) -> (element=w601:i32)
                n438 = Reshape Array(w595, w601) -> (w594:string[])
                n439 = Search 1D Array(1D array=w594, element=w602) -> (index of element=w605:i32)  [unwired: 1 in]
                n440 = Equal?(x=w605, y=-1) -> (x = y?=w604:bool)
                n441 = case shown="True" w604 {
                  tunnel: w593 -> [w615 w624]
                  tunnel: w605 -> [w612 _]
                  tunnel: [w611 w625] -> w603
                  tunnel: w594 -> [_ w622]
                  tunnel: w602 -> [_ w620]
                  frame False {
                    n442 = local read "Re-Calculated Values Cluster"() -> (w608:T9)
                    n443 = Divide(x=w612, y=3) -> (x/y=w614:dbl)
                    n444 = Unbundle By Name(w608) -> ("On/Off"=w607:dbl)
                    n445 = To Word Integer(number=w614) -> (16bit integer=w613:i16)
                    n446 = Format Value(format string="%#g", value (0)=w607) -> (output string=w609:string)  [unwired: 1 in]
                    n447 = Replace Array Subset(array=w615, new element=w609, index (row)=w613, index (col)=1) -> (w611:string[][])
                  }
                  frame True {
                    n448 = local read "Re-Calculated Values Cluster"() -> (w619:T9)
                    n449 = Unbundle By Name(w619) -> ("On/Off"=w618:dbl)
                    n450 = Search 1D Array(1D array=w622, element="On/Off Current:") -> (index of element=w628:i32)  [unwired: 1 in]
                    n451 = Divide(x=w628, y=3) -> (x/y=w629:dbl)
                    n452 = To Word Integer(number=w629) -> (16bit integer=w621:i16)
                    n453 = Format Value(format string="%#g", value (0)=w618) -> (output string=w623:string)  [unwired: 1 in]
                    n454 = Build Array(w620, w623) -> (w627:string[])
                    n455 = Replace Array Subset(array=w624, new element=w627, index (row)=w621) -> (w625:string[][])  [unwired: 1 in]
                  }
                }
                n456 = local write "Save Array"(w603) -> ()
              }
              frame #8 {
                w641 = "Off I-Sat (A):"
                n457 = local read "Save Array"() -> (w632:string[][])
                n458 = Array Size(array=w632) -> (size(s)=w638:i32[])
                n459 = Array Subset(array=w632, index (row)=0, index (col)=0, length (col)=3) -> (w634:string[][])  [unwired: 1 in]
                n460 = Index Array(array=w638, index=0) -> (element=w640:i32)
                n461 = Reshape Array(w634, w640) -> (w633:string[])
                n462 = Search 1D Array(1D array=w633, element=w641) -> (index of element=w644:i32)  [unwired: 1 in]
                n463 = Equal?(x=w644, y=-1) -> (x = y?=w643:bool)
                n464 = case shown="True" w643 {
                  tunnel: w632 -> [w654 w662]
                  tunnel: w644 -> [w651 _]
                  tunnel: [w650 w661] -> w642
                  tunnel: w633 -> [_ w660]
                  tunnel: w641 -> [_ w659]
                  frame False {
                    n465 = local read "Re-Calculated Values Cluster"() -> (w647:T9)
                    n466 = Unbundle By Name(w647) -> ("Off Current"=w646:dbl)
                    n467 = Divide(x=w651, y=3) -> (x/y=w653:dbl)
                    n468 = Format Value(format string="%#g", value (0)=w646) -> (output string=w648:string)  [unwired: 1 in]
                    n469 = To Word Integer(number=w653) -> (16bit integer=w652:i16)
                    n470 = Replace Array Subset(array=w654, new element=w648, index (row)=w652, index (col)=1) -> (w650:string[][])
                  }
                  frame True {
                    n471 = local read "Re-Calculated Values Cluster"() -> (w658:T9)
                    n472 = Unbundle By Name(w658) -> ("Off Current"=w657:dbl)
                    n473 = Search 1D Array(1D array=w660, element="On/Off I-Sat:") -> (index of element=w667:i32)  [unwired: 1 in]
                    n474 = Divide(x=w667, y=3) -> (x/y=w668:dbl)
                    n475 = To Word Integer(number=w668) -> (16bit integer=w666:i16)
                    n476 = Format Value(format string="%#g", value (0)=w657) -> (output string=w671:string)  [unwired: 1 in]
                    n477 = Build Array(w659, w671) -> (w664:string[])
                    n478 = Increment(x=w666) -> (x+1=w665:i16)
                    n479 = Insert Into Array(array=w662, index (row)=w665, new element=w664) -> (w661:string[][])  [unwired: 1 in]
                  }
                }
                n480 = local write "Save Array"(w642) -> ()
              }
              frame #9 {
                w673 = "Vt-Sat (V):"
                n481 = local read "Save Array"() -> (w674:string[][])
                n482 = Array Size(array=w674) -> (size(s)=w679:i32[])
                n483 = Array Subset(array=w674, index (row)=0, index (col)=0, length (col)=3) -> (w675:string[][])  [unwired: 1 in]
                n484 = Index Array(array=w679, index=0) -> (element=w681:i32)
                n485 = Reshape Array(w675, w681) -> (w672:string[])
                n486 = Search 1D Array(1D array=w672, element=w673) -> (index of element=w684:i32)  [unwired: 1 in]
                n487 = Equal?(x=w684, y=-1) -> (x = y?=w683:bool)
                n488 = case shown="False" w683 {
                  tunnel: w674 -> [w693 w703]
                  tunnel: w684 -> [w689 _]
                  tunnel: [w688 w702] -> w682
                  tunnel: w673 -> [_ w701]
                  tunnel: w672 -> [_ w700]
                  frame False {
                    n489 = local read "Re-Calculated Values Cluster"() -> (w687:T9)
                    n490 = Unbundle By Name(w687) -> ("Vt-Sat"=w686:dbl)
                    n491 = Divide(x=w689, y=3) -> (x/y=w692:dbl)
                    n492 = To Word Integer(number=w692) -> (16bit integer=w691:i16)
                    n493 = Number To Fractional String(number=w686) -> (F-format string=w690:string)  [unwired: 3 in]
                    n494 = Replace Array Subset(array=w693, new element=w690, index (row)=w691, index (col)=1) -> (w688:string[][])
                  }
                  frame True {
                    n495 = local read "Re-Calculated Values Cluster"() -> (w697:T9)
                    n496 = Unbundle By Name(w697) -> ("Vt-Sat"=w696:dbl)
                    n497 = Search 1D Array(1D array=w700, element="Threshold V (V):") -> (index of element=w699:i32)  [unwired: 1 in]
                    n498 = Divide(x=w699, y=3) -> (x/y=w706:dbl)
                    n499 = To Word Integer(number=w706) -> (16bit integer=w698:i16)
                    n500 = Format Value(format string="%#g", value (0)=w696) -> (output string=w709:string)  [unwired: 1 in]
                    n501 = Build Array(w701, w709) -> (w705:string[])
                    n502 = Replace Array Subset(array=w703, new element=w705, index (row)=w698) -> (w702:string[][])  [unwired: 1 in]
                  }
                }
                n503 = local write "Save Array"(w682) -> ()
              }
              frame #10 {
                n504 = disable-structure shown="Disabled" {
                  frame Disabled {
                    n505 = local read "Save Array"() -> (w710:string[][])
                    n506 = Array Size(array=w710) -> (size(s)=w716:i32[])
                    n507 = Array Subset(array=w710, index (row)=0, index (col)=0, length (col)=3) -> (w712:string[][])  [unwired: 1 in]
                    n508 = Index Array(array=w716, index=0) -> (element=w718:i32)
                    n509 = Reshape Array(w712, w718) -> (w711:string[])
                    n510 = Search 1D Array(1D array=w711, element="VT-Lin (V):") -> (index of element=w721:i32)  [unwired: 1 in]
                    n511 = Equal?(x=w721, y=-1) -> (x = y?=w720:bool)
                    n512 = case shown="False" w720 {
                      tunnel: w710 -> [w730 w733]
                      tunnel: w721 -> [w727 _]
                      tunnel: [w726 w733] -> w719
                      frame False {
                        n513 = Divide(x=w727, y=3) -> (x/y=w729:dbl)
                        n514 = To Word Integer(number=w729) -> (16bit integer=w728:i16)
                        n515 = Format Value(format string="%#g") -> (output string=w724:string)  [unwired: 2 in]
                        n516 = Replace Array Subset(array=w730, new element=w724, index (row)=w728, index (col)=1) -> (w726:string[][])
                      }
                      frame True {
                      }
                    }
                    n517 = local write "Save Array"(w719) -> ()
                  }
                  frame Enabled {
                  }
                }
              }
              frame #11 {
                w734 = "STS-Sat (V/decade):"
                n518 = local read "Save Array"() -> (w736:string[][])
                n519 = Array Size(array=w736) -> (size(s)=w741:i32[])
                n520 = Array Subset(array=w736, index (row)=0, index (col)=0, length (col)=3) -> (w737:string[][])  [unwired: 1 in]
                n521 = Index Array(array=w741, index=0) -> (element=w743:i32)
                n522 = Reshape Array(w737, w743) -> (w735:string[])
                n523 = Search 1D Array(1D array=w735, element=w734) -> (index of element=w746:i32)  [unwired: 1 in]
                n524 = Equal?(x=w746, y=-1) -> (x = y?=w745:bool)
                n525 = case shown="True" w745 {
                  tunnel: w736 -> [w756 w764]
                  tunnel: w746 -> [w753 _]
                  tunnel: [w752 w765] -> w744
                  tunnel: w735 -> [_ w763]
                  tunnel: w734 -> [_ w762]
                  frame False {
                    n526 = local read "Re-Calculated Values Cluster"() -> (w748:T9)
                    n527 = Unbundle By Name(w748) -> ("STS"=w749:dbl)
                    n528 = Divide(x=w753, y=3) -> (x/y=w755:dbl)
                    n529 = To Word Integer(number=w755) -> (16bit integer=w754:i16)
                    n530 = Format Value(format string="%#g", value (0)=w749) -> (output string=w750:string)  [unwired: 1 in]
                    n531 = Replace Array Subset(array=w756, new element=w750, index (row)=w754, index (col)=1) -> (w752:string[][])
                  }
                  frame True {
                    n532 = local read "Re-Calculated Values Cluster"() -> (w759:T9)
                    n533 = Unbundle By Name(w759) -> ("STS"=w760:dbl)
                    n534 = Search 1D Array(1D array=w763, element="S.T.S. (V/decade):") -> (index of element=w768:i32)  [unwired: 1 in]
                    n535 = Divide(x=w768, y=3) -> (x/y=w769:dbl)
                    n536 = To Word Integer(number=w769) -> (16bit integer=w761:i16)
                    n537 = Format Value(format string="%#g", value (0)=w760) -> (output string=w772:string)  [unwired: 1 in]
                    n538 = Build Array(w762, w772) -> (w767:string[])
                    n539 = Replace Array Subset(array=w764, new element=w767, index (row)=w761) -> (w765:string[][])  [unwired: 1 in]
                  }
                }
                n540 = local write "Save Array"(w744) -> ()
              }
              frame #12 {
                w773 = "Trap Density-VT (Traps/Vcm^2):"
                n541 = local read "Save Array"() -> (w775:string[][])
                n542 = Array Size(array=w775) -> (size(s)=w780:i32[])
                n543 = Array Subset(array=w775, index (row)=0, index (col)=0, length (col)=3) -> (w776:string[][])  [unwired: 1 in]
                n544 = Index Array(array=w780, index=0) -> (element=w782:i32)
                n545 = Reshape Array(w776, w782) -> (w774:string[])
                n546 = Search 1D Array(1D array=w774, element=w773) -> (index of element=w785:i32)  [unwired: 1 in]
                n547 = Equal?(x=w785, y=-1) -> (x = y?=w784:bool)
                n548 = case shown="True" w784 {
                  tunnel: w775 -> [w795 w802]
                  tunnel: w785 -> [w791 _]
                  tunnel: [w790 w803] -> w783
                  tunnel: w774 -> [_ w801]
                  tunnel: w773 -> [_ w800]
                  frame False {
                    n549 = local read "Re-Calculated Values Cluster"() -> (w788:T9)
                    n550 = Unbundle By Name(w788) -> ("Trap Density-VT"=w787:dbl)
                    n551 = Divide(x=w791, y=3) -> (x/y=w794:dbl)
                    n552 = To Word Integer(number=w794) -> (16bit integer=w793:i16)
                    n553 = Format Value(format string="%#g", value (0)=w787) -> (output string=w792:string)  [unwired: 1 in]
                    n554 = Replace Array Subset(array=w795, new element=w792, index (row)=w793, index (col)=1) -> (w790:string[][])
                  }
                  frame True {
                    n555 = local read "Re-Calculated Values Cluster"() -> (w799:T9)
                    n556 = Unbundle By Name(w799) -> ("Trap Density-VT"=w798:dbl)
                    n557 = Search 1D Array(1D array=w801, element="STS-Sat (V/decade):") -> (index of element=w808:i32)  [unwired: 1 in]
                    n558 = Divide(x=w808, y=3) -> (x/y=w807:dbl)
                    n559 = To Word Integer(number=w807) -> (16bit integer=w809:i16)
                    n560 = Format Value(format string="%#g", value (0)=w798) -> (output string=w804:string)  [unwired: 1 in]
                    n561 = Build Array(w800, w804) -> (w811:string[])
                    n562 = Increment(x=w809) -> (x+1=w810:i16)
                    n563 = Insert Into Array(array=w802, index (row)=w810, new element=w811) -> (w803:string[][])  [unwired: 1 in]
                  }
                }
                n564 = local write "Save Array"(w783) -> ()
              }
              frame #13 {
                w813 = "Trap Density-STS (Traps/Vcm^2):"
                n565 = local read "Save Array"() -> (w815:string[][])
                n566 = Array Size(array=w815) -> (size(s)=w820:i32[])
                n567 = Array Subset(array=w815, index (row)=0, index (col)=0, length (col)=3) -> (w816:string[][])  [unwired: 1 in]
                n568 = Index Array(array=w820, index=0) -> (element=w822:i32)
                n569 = Reshape Array(w816, w822) -> (w814:string[])
                n570 = Search 1D Array(1D array=w814, element=w813) -> (index of element=w825:i32)  [unwired: 1 in]
                n571 = Equal?(x=w825, y=-1) -> (x = y?=w824:bool)
                n572 = case shown="True" w824 {
                  tunnel: w815 -> [w835 w842]
                  tunnel: w825 -> [w832 _]
                  tunnel: [w831 w843] -> w823
                  tunnel: w814 -> [_ w841]
                  tunnel: w813 -> [_ w840]
                  frame False {
                    n573 = local read "Re-Calculated Values Cluster"() -> (w828:T9)
                    n574 = Unbundle By Name(w828) -> ("Trap Density-STS"=w827:dbl)
                    n575 = Divide(x=w832, y=3) -> (x/y=w834:dbl)
                    n576 = To Word Integer(number=w834) -> (16bit integer=w833:i16)
                    n577 = Format Value(format string="%#g", value (0)=w827) -> (output string=w829:string)  [unwired: 1 in]
                    n578 = Replace Array Subset(array=w835, new element=w829, index (row)=w833, index (col)=1) -> (w831:string[][])
                  }
                  frame True {
                    n579 = local read "Re-Calculated Values Cluster"() -> (w839:T9)
                    n580 = Unbundle By Name(w839) -> ("Trap Density-STS"=w838:dbl)
                    n581 = Search 1D Array(1D array=w841, element="Trap Density-VT (Traps/Vcm^2):") -> (index of element=w848:i32)  [unwired: 1 in]
                    n582 = Divide(x=w848, y=3) -> (x/y=w849:dbl)
                    n583 = To Word Integer(number=w849) -> (16bit integer=w847:i16)
                    n584 = Format Value(format string="%#g", value (0)=w838) -> (output string=w852:string)  [unwired: 1 in]
                    n585 = Build Array(w840, w852) -> (w845:string[])
                    n586 = Increment(x=w847) -> (x+1=w846:i16)
                    n587 = Insert Into Array(array=w842, index (row)=w846, new element=w845) -> (w843:string[][])  [unwired: 1 in]
                  }
                }
                n588 = local write "Save Array"(w823) -> ()
              }
            }
            n589 = local read "New: Temp"() -> (w360:dbl)
            n590 = local read "New: Width"() -> (w361:dbl)
            n591 = local read "New: Length"() -> (w363:dbl)
            n592 = local read "Index"() -> (w362:string)
            n593 = To Single Precision Float(number=w360) -> (single precision float=w377:sgl)
            n594 = Number To Decimal String(number=w377) -> (decimal integer string=w372:string)  [unwired: 1 in]
            n595 = To Single Precision Float(number=w361) -> (single precision float=w376:sgl)
            n596 = To Single Precision Float(number=w363) -> (single precision float=w375:sgl)
            n597 = Strip Path(path=w359) -> (stripped path=w364:path)  [unwired: 1 out]
            n598 = Number To Decimal String(number=w375) -> (decimal integer string=w370:string)  [unwired: 1 in]
            n599 = Number To Decimal String(number=w376) -> (decimal integer string=w369:string)  [unwired: 1 in]
            n600 = Concatenate Strings("_", w372, "K") -> (w374:string)
            n601 = call "Build Text"("Temp"=w374, "Index"=w362, "Length"=w370, "Width"=w369) -> ("Result"=w368:string)  [unwired: 10 in, 1 out]
            n602 = Path To String(path=w364) -> (string=w366:string)
            n603 = Concatenate Strings(w366, "\\", w368) -> (w367:string)
            n604 = String To Path(string=w367) -> (path=w358:path)
          }
          frame #1 {
            n605 = flat-sequence {
              tunnel: w856 -> [w858]
              tunnel: w855 -> [w857]
              tunnel: [w857] -> w854
              tunnel: w854 -> [w864]
              tunnel: w853 -> [w863]
              frame #0 {
                n606 = Equal?(x=w858, y=w857) -> (x = y?=w859:bool)
                n607 = case shown="False" w859 {
                  tunnel: w858 -> [w862 _]
                  tunnel: w857 -> [w861 _]
                  frame False {
                    n608 = Move(source path=w862, 9:TRUE, 10:w861) -> ()  [unwired: 2 in, 3 out]
                  }
                  frame True {
                  }
                }
              }
              frame #1 {
                n609 = local write "Transfer File"(w864) -> ()
                n610 = call-poly <vilib>:"Write To Spreadsheet File.vi"("2D data"=w863, "file path (dialog if empty)"=w864) -> ()  [unwired: 6 in, 1 out]
              }
            }
          }
        }
        n611 = Cluster To Array(cluster=w348) -> (array=w347:bool[])
        n612 = Boolean Array To Number(Boolean array=w347) -> (number=w346:u32)
        n613 = Equal To 0?(x=w346) -> (x = 0?=w345:bool)
        n614 = case shown="True" w345 {
          tunnel: [MegaAwesome_States."Read Data" w352] -> w344
          tunnel: w343 -> [_ w356]
          frame False {
          }
          frame True {
            n615 = Unbundle By Name(w356) -> ("Save Next"=w355:bool)
            n616 = Select(t=MegaAwesome_States."No Event", s=w355, f=MegaAwesome_States."Next File") -> (s? t:f=w352:T2)
          }
        }
      }
      frame "Exit" {
      }
      frame "Save Lines" {
      }
      frame "Export" {
        n617 = flat-sequence {
          frame #0 {
            n618 = stacked-sequence {
              frame #0 {
                n619 = local read "Independant Variable:"() -> (w871:string)
                n620 = Equal?(x=w871, y="Length (um):") -> (x = y?=w872:bool)
                n621 = case shown="True" w872 {
                  frame False {
                  }
                  frame True {
                    n622 = local write "X Axis Display Type"("1") -> ()
                    n623 = local write "Opj X Axis"("2") -> ()
                  }
                }
              }
              frame #1 {
                n624 = local read "Independant Variable:"() -> (w876:string)
                n625 = Equal?(x=w876, y="Sample Temp (K):") -> (x = y?=w877:bool)
                n626 = case shown="True" w877 {
                  frame False {
                  }
                  frame True {
                    n627 = local write "X Axis Display Type"("1") -> ()
                    n628 = local write "Opj X Axis"("1") -> ()
                  }
                }
              }
              frame #2 {
                n629 = local read "Independant Variable:"() -> (w881:string)
                n630 = Equal?(x=w881, y="Mobility-Sat (cm^2/Vs):") -> (x = y?=w882:bool)
                n631 = case shown="True" w882 {
                  frame False {
                  }
                  frame True {
                    n632 = local write "X Axis Display Type"("2") -> ()
                    n633 = local write "Opj X Axis"("2") -> ()
                  }
                }
              }
              frame #3 {
                n634 = local read "Independant Variable:"() -> (w886:string)
                n635 = Equal?(x=w886, y="Mobility-Lin (cm^2/Vs):") -> (x = y?=w887:bool)
                n636 = case shown="True" w887 {
                  frame False {
                  }
                  frame True {
                    n637 = local write "X Axis Display Type"("2") -> ()
                    n638 = local write "Opj X Axis"("2") -> ()
                  }
                }
              }
              frame #4 {
                n639 = local read "Independant Variable:"() -> (w891:string)
                n640 = Equal?(x=w891, y="On/Off I-Sat:") -> (x = y?=w892:bool)
                n641 = case shown="True" w892 {
                  frame False {
                  }
                  frame True {
                    n642 = local write "X Axis Display Type"("2") -> ()
                    n643 = local write "Opj X Axis"("2") -> ()
                  }
                }
              }
              frame #5 {
                n644 = local read "Independant Variable:"() -> (w896:string)
                n645 = Equal?(x=w896, y="Off I-Sat (A):") -> (x = y?=w897:bool)
                n646 = case shown="True" w897 {
                  frame False {
                  }
                  frame True {
                    n647 = local write "X Axis Display Type"("2") -> ()
                    n648 = local write "Opj X Axis"("2") -> ()
                  }
                }
              }
              frame #6 {
                n649 = local read "Independant Variable:"() -> (w901:string)
                n650 = Equal?(x=w901, y="Vt-Sat (V):") -> (x = y?=w902:bool)
                n651 = case shown="True" w902 {
                  frame False {
                  }
                  frame True {
                    n652 = local write "X Axis Display Type"("1") -> ()
                    n653 = local write "Opj X Axis"("1") -> ()
                  }
                }
              }
              frame #7 {
                n654 = local read "Independant Variable:"() -> (w906:string)
                n655 = Equal?(x=w906, y="STS-Sat (V/decade):") -> (x = y?=w907:bool)
                n656 = case shown="True" w907 {
                  frame False {
                  }
                  frame True {
                    n657 = local write "X Axis Display Type"("1") -> ()
                    n658 = local write "Opj X Axis"("1") -> ()
                  }
                }
              }
              frame #8 {
                n659 = local read "Independant Variable:"() -> (w911:string)
                n660 = Equal?(x=w911, y="Trap Density-VT (Traps/Vcm^2):") -> (x = y?=w912:bool)
                n661 = case shown="True" w912 {
                  frame False {
                  }
                  frame True {
                    n662 = local write "X Axis Display Type"("2") -> ()
                    n663 = local write "Opj X Axis"("2") -> ()
                  }
                }
              }
              frame #9 {
                n664 = local read "Independant Variable:"() -> (w916:string)
                n665 = Equal?(x=w916, y="Trap Density-STS (Traps/Vcm^2):") -> (x = y?=w917:bool)
                n666 = case shown="True" w917 {
                  frame False {
                  }
                  frame True {
                    n667 = local write "X Axis Display Type"("2") -> ()
                    n668 = local write "Opj X Axis"("2") -> ()
                  }
                }
              }
            }
          }
          frame #1 {
            n669 = local read "Transfer Folder"() -> (w925:path)
            n670 = Build Path(base path=w925, name or relative path="Stats") -> (appended path=w926:path)
            n671 = local read "Origin Project File"() -> (w937:path)
            n672 = call <vilib>:"Check if File or Folder Exists.vi"("path"=w926) -> ("file or folder exists?"=w941:bool, "dup path"=w940:path)  [unwired: 8 in, 1 out]
            n673 = call <userlib>:"OA_ConnectToOrigin.vi"() -> ("error out"=w938:errorcluster, "Origin.IOApplication"=w939:refnum<k7>)  [unwired: 8 in]
            n674 = case shown="False" w941 {
              tunnel: w940 -> [w1114 w1115]
              tunnel: [w1113 w1115] -> w924
              frame False {
                n675 = Create Folder(path (use dialog)=w1114) -> (created path=w1113:path)  [unwired: 2 in, 2 out]
              }
              frame True {
              }
            }
            n676 = call "File Dialog"("start path"=w926) -> ("selected path"=w928:path)  [unwired: 11 in, 3 out]
            n677 = call <userlib>:"OA_Load.vi"("error in (no error)"=w938, "Path"=w937, "Origin.IOApplication"=w939) -> ("error out"=w935:errorcluster, "Origin.IOApplication"=w936:refnum<k7>)  [unwired: 1 out]
            n678 = call "OAExecute.vi"("script"="document -m 3;", "Error IO"=w935, "Origin.IOApplication"=w936) -> ("Error IO Out"=w933:errorcluster, "Origin.IOApplication"=w934:refnum<k7>)  [unwired: 1 in, 1 out]
            n679 = local read "Independant Variable:"() -> (w921:string)
            n680 = stacked-sequence {
              tunnel: w925 -> [w952 w982 w994 w1016 w1036 w1057 w1078 w1101]
              tunnel: w924 -> [w953 w981 w995 w1015 w1037 w1058 w1079 w1102]
              tunnel: w934 -> [w955 w979 w997 w1018 w1039 w1060 w1081 w1104]
              tunnel: w933 -> [w954 w980 w996 w1017 w1038 w1059 w1080 w1103]
              tunnel: [_ _ _ _ _ _ _ w1099] -> w923
              tunnel: [_ _ _ _ _ _ _ w1100] -> w922
              tunnel: w921 -> [w951 w972 w993 w1014 w1035 w1056 w1077 w1098]
              frame #0 {
                n681 = local read "X Axis Display Type"() -> (w943:string)
                n682 = local read "Opj X Axis"() -> (w948:string)
                n683 = Concatenate Strings("window -a MOBLGraph;\nlayer.x.type=", w948, "; layer.x.label.numFormat = ", w943, "; Y3 = 1; X3 = 1;", "window -a MOBLTable;\nwindow -s TV;") -> (w946:string)
                n684 = call "Param_Analysis_7_24b_JW.vi"("Independant Variable"=w951, "error in (no error)"=w954, "Data Folder"=w952, "Parameter String"="Mobility-Lin (cm^2/Vs):", "Parameter Name"="Mobility-Lin", "Stats Folder"=w953) -> ("error out"=w957:errorcluster, "Output Array"=w959:string[][], "Variables"=w950:T16)  [unwired: 2 in, 1 out]
                n685 = call "Origin_Export_7_27a_JW.vi"("Input Conditions"=w950, "Analysis Array"=w959, "error in (no error)"=w957, "Parameter Worksheet Name"="[MOBLTable]Mobilities", "Parameter Folder Script"="pe_cd \"Mobility-Lin\";", "Origin.IOApplication"=w955) -> ("error out"=w956:errorcluster, "reference out"=w958:refnum<k7>)  [unwired: 3 in, 1 out]
                n686 = call "OAExecute.vi"("script"=w946, "Error IO"=w956, "Origin.IOApplication"=w958) -> ()  [unwired: 1 in, 3 out]
              }
              frame #1 {
                n687 = local read "X Axis Display Type"() -> (w964:string)
                n688 = local read "Opj X Axis"() -> (w969:string)
                n689 = Concatenate Strings("window -a MOBSGraph;\nlayer.x.type=", w969, "; layer.x.label.numFormat = ", w964, "; Y3 = 1; X3 = 1;", "window -a MOBSTable;\nwindow -s TV;") -> (w967:string)
                n690 = call "Param_Analysis_7_24b_JW.vi"("Independant Variable"=w972, "error in (no error)"=w980, "Data Folder"=w982, "Parameter String"="Mobility-Sat (cm^2/Vs):", "Parameter Name"="Mobility-Sat", "Stats Folder"=w981) -> ("error out"=w975:errorcluster, "Output Array"=w973:string[][], "Variables"=w971:T16)  [unwired: 2 in, 1 out]
                n691 = call "Origin_Export_7_27a_JW.vi"("Input Conditions"=w971, "Analysis Array"=w973, "error in (no error)"=w975, "Parameter Worksheet Name"="[MOBSTable]Mobilities", "Parameter Folder Script"="pe_cd \"Mobility-Sat\";", "Origin.IOApplication"=w979) -> ("error out"=w974:errorcluster, "reference out"=w976:refnum<k7>)  [unwired: 3 in, 1 out]
                n692 = call "OAExecute.vi"("script"=w967, "Error IO"=w974, "Origin.IOApplication"=w976) -> ()  [unwired: 1 in, 3 out]
              }
              frame #2 {
                n693 = local read "X Axis Display Type"() -> (w985:string)
                n694 = local read "Opj X Axis"() -> (w990:string)
                n695 = Concatenate Strings("window -a NSTSGraph;\nlayer.x.type=", w990, "; layer.x.label.numFormat = ", w985, "; Y3 = 1; X3 = 1;", "window -a NSTSTable;\nwindow -s TV;") -> (w988:string)
                n696 = call "Param_Analysis_7_24b_JW.vi"("Independant Variable"=w993, "error in (no error)"=w996, "Data Folder"=w994, "Parameter String"="Trap Density-STS (Traps/Vcm^2):", "Parameter Name"="Trap Density-STS", "Stats Folder"=w995) -> ("error out"=w1000:errorcluster, "Output Array"=w998:string[][], "Variables"=w992:T16)  [unwired: 2 in, 1 out]
                n697 = call "Origin_Export_7_27a_JW.vi"("Input Conditions"=w992, "Analysis Array"=w998, "error in (no error)"=w1000, "Parameter Worksheet Name"="[NSTSTable]Trap Densities", "Parameter Folder Script"="pe_cd \"N-STS\";", "Origin.IOApplication"=w997) -> ("error out"=w999:errorcluster, "reference out"=w1001:refnum<k7>)  [unwired: 3 in, 1 out]
                n698 = call "OAExecute.vi"("script"=w988, "Error IO"=w999, "Origin.IOApplication"=w1001) -> ()  [unwired: 1 in, 3 out]
              }
              frame #3 {
                n699 = local read "X Axis Display Type"() -> (w1006:string)
                n700 = local read "Opj X Axis"() -> (w1011:string)
                n701 = call "Param_Analysis_7_24b_JW.vi"("Independant Variable"=w1014, "error in (no error)"=w1017, "Data Folder"=w1016, "Parameter String"="Trap Density-VT (Traps/Vcm^2):", "Parameter Name"="Trap Density-Vt", "Stats Folder"=w1015) -> ("error out"=w1021:errorcluster, "Output Array"=w1019:string[][], "Variables"=w1013:T16)  [unwired: 2 in, 1 out]
                n702 = Concatenate Strings("window -a NVtGraph;\nlayer.x.type=", w1011, "; layer.x.label.numFormat = ", w1006, "; Y3 = 1; X3 = 1;", "window -a NVtTable;\nwindow -s TV;") -> (w1009:string)
                n703 = call "Origin_Export_7_27a_JW.vi"("Input Conditions"=w1013, "Analysis Array"=w1019, "error in (no error)"=w1021, "Parameter Worksheet Name"="[NVTTable]Trap Densities", "Parameter Folder Script"="pe_cd \"N-Vt\";", "Origin.IOApplication"=w1018) -> ("error out"=w1020:errorcluster, "reference out"=w1022:refnum<k7>)  [unwired: 3 in, 1 out]
                n704 = call "OAExecute.vi"("script"=w1009, "Error IO"=w1020, "Origin.IOApplication"=w1022) -> ()  [unwired: 1 in, 3 out]
              }
              frame #4 {
                n705 = local read "X Axis Display Type"() -> (w1027:string)
                n706 = local read "Opj X Axis"() -> (w1032:string)
                n707 = Concatenate Strings("window -a OffIGraph;\nlayer.x.type=", w1032, "; layer.x.label.numFormat = ", w1027, "; Y3 = 1; X3 = 1;", "window -a OffITable;\nwindow -s TV;") -> (w1030:string)
                n708 = call "Param_Analysis_7_24b_JW.vi"("Independant Variable"=w1035, "error in (no error)"=w1038, "Data Folder"=w1036, "Parameter String"="Off I-Sat (A):", "Parameter Name"="Off I-Sat", "Stats Folder"=w1037) -> ("error out"=w1042:errorcluster, "Output Array"=w1040:string[][], "Variables"=w1034:T16)  [unwired: 2 in, 1 out]
                n709 = call "Origin_Export_7_27a_JW.vi"("Input Conditions"=w1034, "Analysis Array"=w1040, "error in (no error)"=w1042, "Parameter Worksheet Name"="[OffItable]OffCurrents", "Parameter Folder Script"="pe_cd \"OffI-Sat\";", "Origin.IOApplication"=w1039) -> ("error out"=w1041:errorcluster, "reference out"=w1043:refnum<k7>)  [unwired: 3 in, 1 out]
                n710 = call "OAExecute.vi"("script"=w1030, "Error IO"=w1041, "Origin.IOApplication"=w1043) -> ()  [unwired: 1 in, 3 out]
              }
              frame #5 {
                n711 = local read "X Axis Display Type"() -> (w1048:string)
                n712 = local read "Opj X Axis"() -> (w1053:string)
                n713 = Concatenate Strings("window -a OnOffGraph;\nlayer.x.type=", w1053, "; layer.x.label.numFormat = ", w1048, "; Y3 = 1; X3 = 1;", "window -a OnOffTable;\nwindow -s TV;") -> (w1051:string)
                n714 = call "Param_Analysis_7_24b_JW.vi"("Independant Variable"=w1056, "error in (no error)"=w1059, "Data Folder"=w1057, "Parameter String"="On/Off I-Sat:", "Parameter Name"="OnOff Ratio", "Stats Folder"=w1058) -> ("error out"=w1063:errorcluster, "Output Array"=w1061:string[][], "Variables"=w1055:T16)  [unwired: 2 in, 1 out]
                n715 = call "Origin_Export_7_27a_JW.vi"("Input Conditions"=w1055, "Analysis Array"=w1061, "error in (no error)"=w1063, "Parameter Worksheet Name"="[OnOffTable]On/Off Ratios", "Parameter Folder Script"="pe_cd \"OnOff-Ratio\";", "Origin.IOApplication"=w1060) -> ("error out"=w1062:errorcluster, "reference out"=w1064:refnum<k7>)  [unwired: 3 in, 1 out]
                n716 = call "OAExecute.vi"("script"=w1051, "Error IO"=w1062, "Origin.IOApplication"=w1064) -> ()  [unwired: 1 in, 3 out]
              }
              frame #6 {
                n717 = local read "X Axis Display Type"() -> (w1069:string)
                n718 = local read "Opj X Axis"() -> (w1074:string)
                n719 = call "Param_Analysis_7_24b_JW.vi"("Independant Variable"=w1077, "error in (no error)"=w1080, "Data Folder"=w1078, "Parameter String"="STS-Sat (V/decade):", "Parameter Name"="STS-Sat", "Stats Folder"=w1079) -> ("error out"=w1084:errorcluster, "Output Array"=w1082:string[][], "Variables"=w1076:T16)  [unwired: 2 in, 1 out]
                n720 = Concatenate Strings("window -a SGraph;\nlayer.x.type=", w1074, "; layer.x.label.numFormat = ", w1069, "; Y3 = 1; X3 = 1;", "window -a STable;\nwindow -s TV;") -> (w1072:string)
                n721 = call "Origin_Export_7_27a_JW.vi"("Input Conditions"=w1076, "Analysis Array"=w1082, "error in (no error)"=w1084, "Parameter Worksheet Name"="[STable]Threshold Swing", "Parameter Folder Script"="pe_cd \"STS-Sat\";", "Origin.IOApplication"=w1081) -> ("error out"=w1083:errorcluster, "reference out"=w1085:refnum<k7>)  [unwired: 3 in, 1 out]
                n722 = call "OAExecute.vi"("script"=w1072, "Error IO"=w1083, "Origin.IOApplication"=w1085) -> ()  [unwired: 1 in, 3 out]
              }
              frame #7 {
                n723 = local read "X Axis Display Type"() -> (w1090:string)
                n724 = local read "Opj X Axis"() -> (w1095:string)
                n725 = Concatenate Strings("window -a VtGraph;\nlayer.x.type=", w1095, "; layer.x.label.numFormat = ", w1090, "; Y3 = 1; X3 = 1;", "window -a VtTable;\nwindow -s TV;") -> (w1093:string)
                n726 = call "Param_Analysis_7_24b_JW.vi"("Independant Variable"=w1098, "error in (no error)"=w1103, "Data Folder"=w1101, "Parameter String"="Vt-Sat (V):", "Parameter Name"="Vt-Sat", "Stats Folder"=w1102) -> ("error out"=w1107:errorcluster, "Output Array"=w1105:string[][], "Variables"=w1097:T16)  [unwired: 2 in, 1 out]
                n727 = call "Origin_Export_7_27a_JW.vi"("Input Conditions"=w1097, "Analysis Array"=w1105, "error in (no error)"=w1107, "Parameter Worksheet Name"="[VtTable]Threshold Voltages", "Parameter Folder Script"="pe_cd \"Vt-Sat\";", "Origin.IOApplication"=w1104) -> ("error out"=w1106:errorcluster, "reference out"=w1108:refnum<k7>)  [unwired: 3 in, 1 out]
                n728 = call "OAExecute.vi"("script"=w1093, "Error IO"=w1106, "Origin.IOApplication"=w1108) -> ("Error IO Out"=w1099:errorcluster, "Origin.IOApplication"=w1100:refnum<k7>)  [unwired: 1 in, 1 out]
              }
            }
            n729 = Path To String(path=w928) -> (string=w927:string)
            n730 = call "OAExecute.vi"("script"="pe_cd /; ", "Error IO"=w923, "Origin.IOApplication"=w922) -> ("Error IO Out"=w929:errorcluster, "Origin.IOApplication"=w930:refnum<k7>)  [unwired: 1 in, 1 out]
            n731 = call <userlib>:"OASaveProject.vi"("path"=w927, "Error IO"=w929, "Origin.IOApplication"=w930) -> ()  [unwired: 3 out]
          }
        }
      }
    }
    "Current State" <- w14
    "Folder Index" <- w7
    n732 = Equal?(x=w16, y=MegaAwesome_States."Exit") -> (x = y?=w17:bool)
    n733 = Wait (ms)(milliseconds to wait=10) -> ()  [unwired: 1 out]
  }
